vi "BStAT_(Singles) Update.vi"() -> ()   [LabVIEW 2014]
uses:
  <vilib>/vision/Image Controls.llb/IMAQ Image.ctl
  <vilib>/Utility/file.llb/Read From Spreadsheet File (string).vi
  <vilib>/Utility/file.llb/Read From Spreadsheet File (I64).vi
panel:
  out "Main tab 2":T1(ring)
  in  "fast rewind":bool
  out "refnum of data save file":refnum<file>
  in  "START":bool
  out "frames to write":i64[][](array[numeric])
  in  "Data file":path caption="Data"
  in  "playback speed":dbl(slide)=1.0 min=0.25 max=1.5 step=0.25 scale=0.25..1.5
  in  "Main tab":enum32{"Coding", "Display"}(tab)
  in  "Switch position":bool
  in  "Link Errors":bool
  in  "Player 2":bool
  in  "Player 1":bool
  in  "TC 3":bool
  in  "TR 3":bool
  in  "ML 3":bool
  in  "MC 3":bool
  in  "MR  3":bool
  in  "BC 3":bool
  in  "BL 3":bool
  in  "BR 3":bool
  in  "TL 3":bool
  in  "TC 2":bool
  in  "TR 2":bool
  in  "ML 2":bool
  in  "MC 2":bool
  in  "MR  2":bool
  in  "BC 2":bool
  in  "BL 2":bool
  in  "BR 2":bool
  in  "TL 2":bool
  in  "E2":bool
  in  "E1":bool
  in  "W2":bool
  in  "W1":bool
  in  "P2":i32
  in  "P1":i32
  in  "1 6":bool
  in  "2 6":bool
  in  "3 6":bool
  in  "4 6":bool
  in  "5 6":bool
  in  "6 6":bool
  in  "7 6":bool
  in  "8 6":bool
  in  "1 5":bool
  in  "2 5":bool
  in  "3 5":bool
  in  "4 5":bool
  in  "5 5":bool
  in  "6 5":bool
  in  "7 5":bool
  in  "8 5":bool
  in  "8 3":bool
  in  "7 3":bool
  in  "6 3":bool
  in  "5 3":bool
  in  "4 3":bool
  in  "3 3":bool
  in  "2 3":bool
  in  "1 3":bool
  in  "8 4":bool
  in  "7 4":bool
  in  "6 4":bool
  in  "5 4":bool
  in  "4 4":bool
  in  "3 4":bool
  in  "2 4":bool
  in  "1 4":bool
  in  "1 2":bool
  in  "2 2":bool
  in  "3 2":bool
  in  "4 2":bool
  in  "5 2":bool
  in  "6 2":bool
  in  "7 2":bool
  in  "8 2":bool
  in  "5":bool
  in  "6":bool
  in  "7":bool
  in  "8":bool
  in  "1":bool
  in  "2":bool
  in  "3":bool
  in  "4":bool
  in  "S1":bool
  in  "S2":bool
  in  "1 7":bool
  in  "2 7":bool
  in  "3 7":bool
  in  "4 7":bool
  in  "Code lag(s)":dbl=1.0 min=0.0 max=5.0 step=0.5 format="%#.1g"
  in  "Pause lag(s)":dbl=1.0 min=0.0 max=2.0 step=0.5 format="%#.1g"
  in  "Pause lag on":bool
  in  "Btn 5":string
  in  "Btn 4":string
  in  "Btn 3":string
  in  "Btn 2":string
  in  "Btn 1":string
  in  "Button 1":bool
  in  "Button 5":bool
  in  "Button 4":bool
  in  "Button 3":bool
  in  "Button 2":bool
  in  "Display tab":enum32{"Edit ", "Data Display", "Momentum"}(tab)
  in  "Combine":bool
  out "Btn 6":string
  out "Btn 7":string
  out "Btn 8":string
  out "Btn 9":string
  out "Btn 10":string
  in  "Button 6":bool
  in  "Button 10":bool
  in  "Button 9":bool
  in  "Button 8":bool
  in  "Button 7":bool
  in  "ST":bool
  in  "CR 2":bool
  in  "player2":bool
  in  "player1":bool
  in  "REPORT":bool
  out "Video files to write":string[](array[string])
  in  "Video compress":bool=TRUE
  in  "Abort":bool
  in  "Write file":bool
  in  "Delete":bool[](array[boolean])
  out "Writing":u32(slide) scale=0.0..51.0
  in  "File name":string
  in  "Add to lib":bool
  in  "Video to write":path caption="Folder"
  in  "Examine code":bool
  in  "Update":bool
  in  "Reset":bool
  in  "Code number display":i32 min=1 max=20
  in  "Next":bool
  in  "Previous":bool
  in  "lob":bool
  in  "clear":bool
  in  "drive":bool
  in  "smash":bool
  in  "defense":bool
  in  "chop":bool
  in  "drop":bool
  in  "net":bool
  in  "FH 2":bool
  in  "BH 2":bool
  in  "OH 2":bool
  in  "after":u8(slide)=2 scale=0.0..5.0
  in  "before":u8(slide)=2
  in  "point 2":bool
  in  "error":bool
  in  "winner":bool
  in  "point 1":bool
  in  "1 9":bool
  in  "service2":bool
  in  "service1":bool
  in  "2 9":bool
  in  "3 8":bool
  in  "4 8":bool
  in  "TL":bool
  in  "BR":bool
  in  "BL":bool
  in  "BM":bool
  in  "CR":bool
  in  "CM":bool
  in  "CL":bool
  in  "TR":bool
  in  "TM":bool
  in  "Extract data":bool
  in  "Upload edited video":bool
  in  "To make white":enum32{""}(tab)
  out "player12":string[](array[string])
  out "player2 2":string[](array[string])
  out "P1graph":cluster{dbl[], "array":dbl[]}(graph)={[0.0, nan, 0.0, nan, 0.0, nan, 0.0, nan, 0.0, nan, 0.0, nan, 0.0, nan, 0.0, nan, 0.0], "array"=[1.0, 2.0, 3.0, 4.0, 5.0, 6.0, 7.0, 8.0, 9.0, 10.0, 11.0, 12.0, 13.0, 14.0, 15.0, 16.0, 17.0]}
  out "P2graph":cluster{dbl[], "array":dbl[]}(graph)={[0.0, nan, 0.0, nan, 0.0, nan, 0.0, nan, 0.0, nan, 0.0, nan, 0.0, nan, 0.0, nan, 0.0], "array"=[1.0, 2.0, 3.0, 4.0, 5.0, 6.0, 7.0, 8.0, 9.0, 10.0, 11.0, 12.0, 13.0, 14.0, 15.0, 16.0, 17.0]}
  out "W1/E1":string[](array[string])
  out "W2/E2":string[](array[string])
  out "W/E2":string[](array[string])=["Fore hand", "Back hand", "Over head", "", "Strainght", "Cross", "", "Lob", "Clear", "Drive", "Smash", "Defence", "Chop", "Drop", "Net"]
  out "W/E1":string[](array[string])=["Fore hand", "Back hand", "Over head", "", "Strainght", "Cross", "", "Lob", "Clear", "Drive", "Smash", "Defence", "Chop", "Drop", "Net"]
  out "player2_2":string[](array[string])
  out "player1_2":string[](array[string])
  out "Player 4":string[](array[string])=["Fore hand", "Back hand", "Over head", "", "Straight", "Cross", "", "Smash", "Defense", "Drive/Tap", "Lob", "Drop", "Chop", "Clear", "Net"]
  out "Player 2_2":string[](array[string])=["Fore hand", "Back hand", "Over head", "", "Strainght", "Cross", "", "Lob", "Clear", "Drive", "Smash", "Defence", "Chop", "Drop", "Net"]
  out "Player 1_2":string[](array[string])=["Fore hand", "Back hand", "Over head", "", "Strainght", "Cross", "", "Lob", "Clear", "Drive", "Smash", "Defence", "Chop", "Drop", "Net"]
  out "Player 3":string[](array[string])=["Fore hand", "Back hand", "Over head", "", "Straight", "Cross", "", "Smash", "Defense", "Drive/Tap", "Lob", "Drop", "Chop", "Clear", "Net"]
  out "p2 17":string
  out "p2 16":string
  out "p2 11":string
  out "p2 10":string
  out "p2 9":string
  out "p2 14":string
  out "p2 13":string
  out "p2 12":string
  out "p2 15":string
  out "p1 5":string
  out "p1 7":string
  out "p1 6":string
  out "p1 4":string
  out "p1 1":string
  out "p1 3":string
  out "p1 2":string
  out "p1 8":string
  out "p1 9":string
  in  "save2":string
  in  "save1":string
  in  "save2 3":bool
  in  "save1 3":bool
  in  "Compare":bool
  in  "2 8":string(combo)="1"
  in  "1 8":string(combo)="1"
  in  "display\nselection":string(combo)="1"
  in  "Percentage":bool
  in  "to make white 2":enum32{""}(tab)
  out "Shortest rally length(sec)":dbl format="%#_3g"
  out "Longest rally length(sec)":dbl format="%#_3g"
  out "Score":dbl[](array[numeric])
  out "Average rally length(sec)":dbl format="%#_3g"
  out "Rally length(sec)":dbl format="%#_3g"
  out "momentum graph":cluster{dbl[], dbl[]}[](graph)
  in  "Load video":bool
  in  "Play":bool
  out "ful video frames":i64[](array[numeric])
  out "playback speed":dbl
  out "Number of Frames":u32
  out "framesPerSecond":u32
  out "Last Edit":bool[](array[boolean])
  out "frames 2 play":i64[](array[numeric])
  in  "stop":bool
  out "Video Frame":u32
  out "save1 2":i32[][](array[numeric])
  out "save1_data":dbl[][](array[numeric])
  out "save2 2":i32[][](array[numeric])
  out "save2_data":dbl[][](array[numeric])
  out "game":i32[][](array[numeric])
  out "comp_p1":dbl[](array[numeric])
  out "comp_p2":dbl[](array[numeric])
  out "comp_p2 2":dbl[](array[numeric])
  out "comp_p1 2":dbl[](array[numeric])
  out "Score 2":i64[][](array[numeric])
  out "frame data":i64[][](array[numeric])
  out "coded data":i64[][](array[numeric])
  out "edited\nevents":i64[][](array[numeric])
  out "edited to play":i64[](array[numeric])
  out "frames edited":i64[](array[numeric])
  out "service frames":i64[](array[numeric])
  out "point frames":i64[](array[numeric])
  out "p1y":dbl[](array[numeric])
  out "p2y":dbl[](array[numeric])
  in  "fast forward":bool
  in  "Pause":bool
  out "coding":i64[][](array[numeric])
  out "FH":bool[](array[boolean])
  out "BH":bool[](array[boolean])
  out "OH":bool[](array[boolean])
  out "P1 position":bool
  out "P2 position":bool
  in  "Progress...":u32(slide) min=400 max=47374 scale=-1.1..47173.0
  in  "Video file":path caption="Video"
  out "task":i32(slide) scale=0.0..300.0
  out "Video":T2(plugin-control)
  # "Strategic Analysis Tool for Badminton"
  # "© 2012 National Sports Institute of Malaysia All Rights Reserved"
  # "Position"
  # "Rally start"
  # "Rally end"
  # "Switch sides"
  # "Smash"
  # "Defence"
  # "Drive/Tap"
  # "Lob"
  # "Drop"
  # "Chop"
  # "Clear"
  # "Net"
  # "Forehand"
  # "Backhand"
  # "Overhead"
  # "Straight"
  # "Cross"
  # "Straight"
  # "Cross"
  # "Straight"
  # "Cross"
  # "Shots"
  # "Custom coding"
  # "Playback interval (s)"
  # "Rally end"
  # "Rally start"
  # "Position"
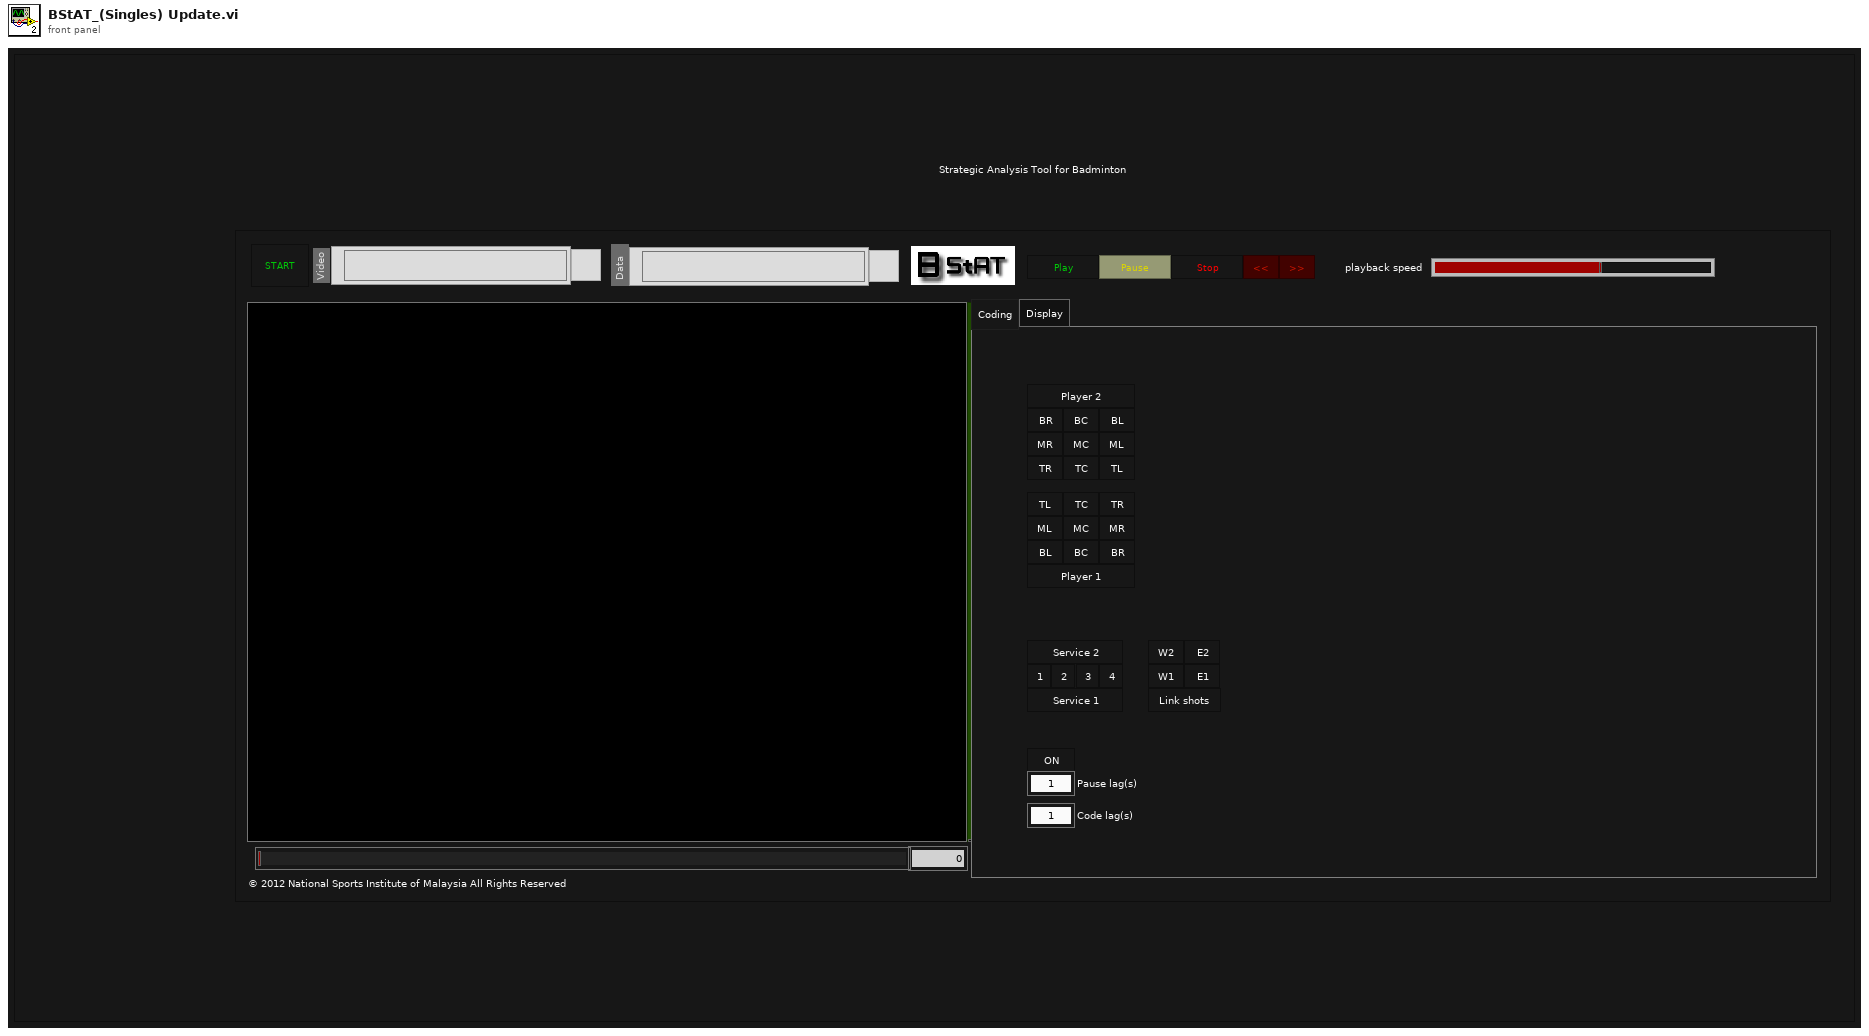
[diagram p1: front panel]
types:
  T1 = enum32{"Coding", "Edit video", "Examine coding", "Display", "Update coding", "Edit coding"}
  T2 = typedef "IMAQ Image.ctl" = refnum<image>
  T3 = enum16{"open", "replace", "create", "open or create", "replace or create", "replace or create with confirmation"}
  T4 = enum8{"Enabled", "Disabled", "Disabled and Grayed Out"}
  T5 = typedef "Image Type" = u32
  T6 = typedef "AviRefnum.ctl" = refnum<k1>
  T7 = cluster{"width":u32, "height":u32, "framesPerSecond":u32, "compressionFilter":string, "hasData":bool}
  T8 = typedef "LVPositionTypeDef.ctl" = cluster{"Left":i32, "Top":i32}
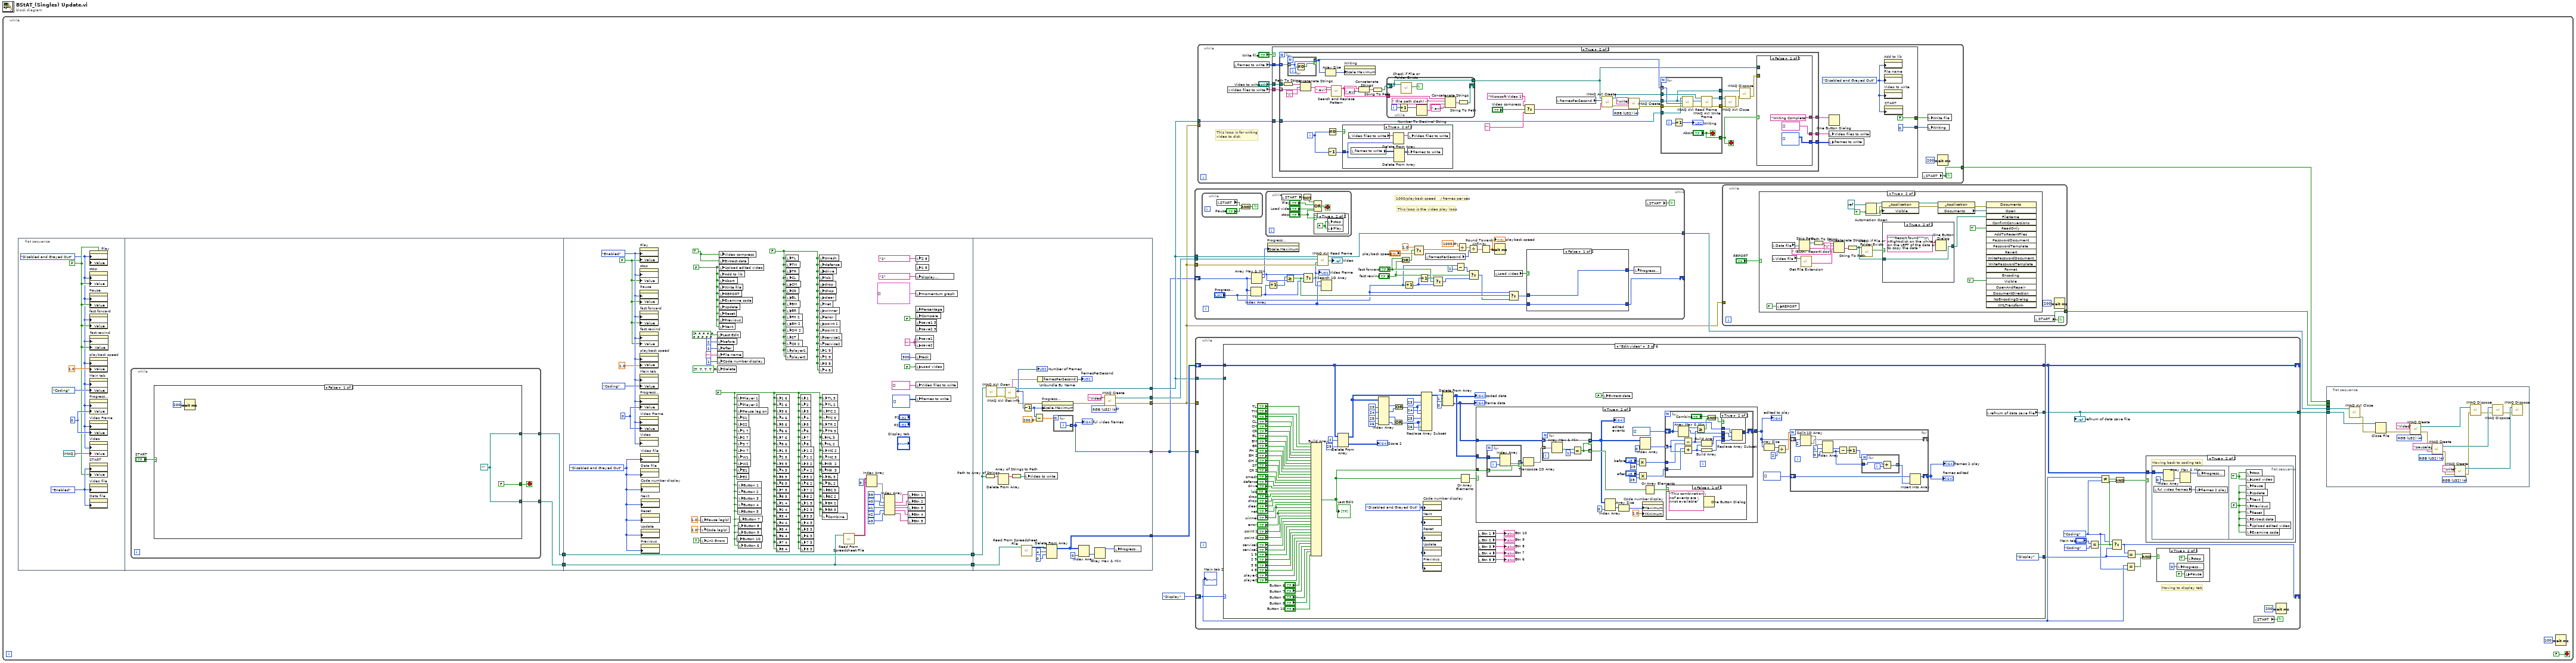
[diagram p0: block diagram]
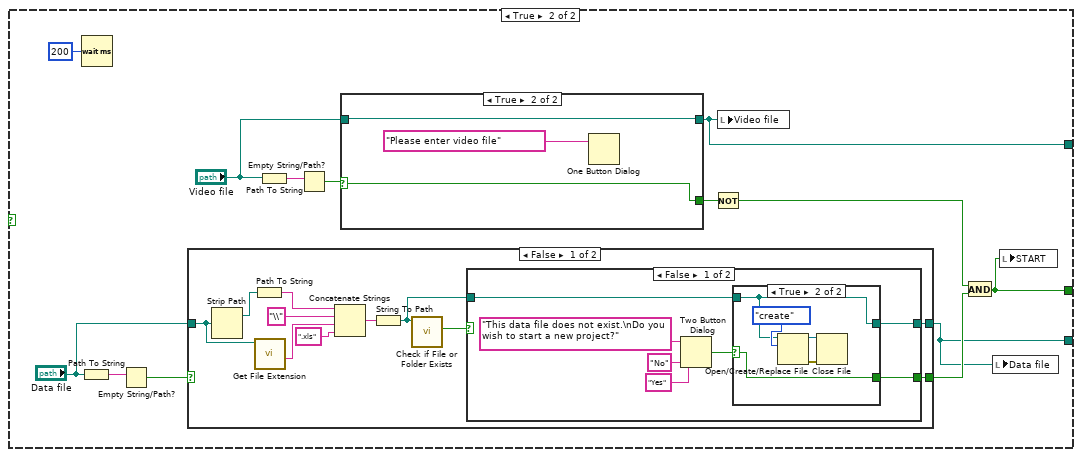
[diagram p2: hidden frame]
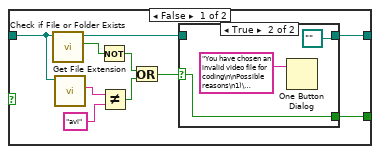
[diagram p3: hidden frame]
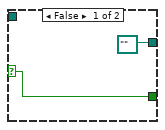
[diagram p5: hidden frame]
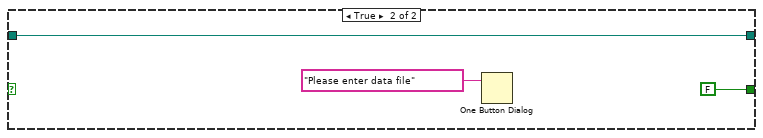
[diagram p7: hidden frame]
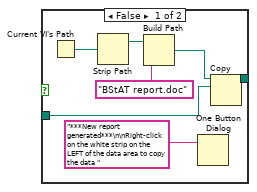
[diagram p9: hidden frame]
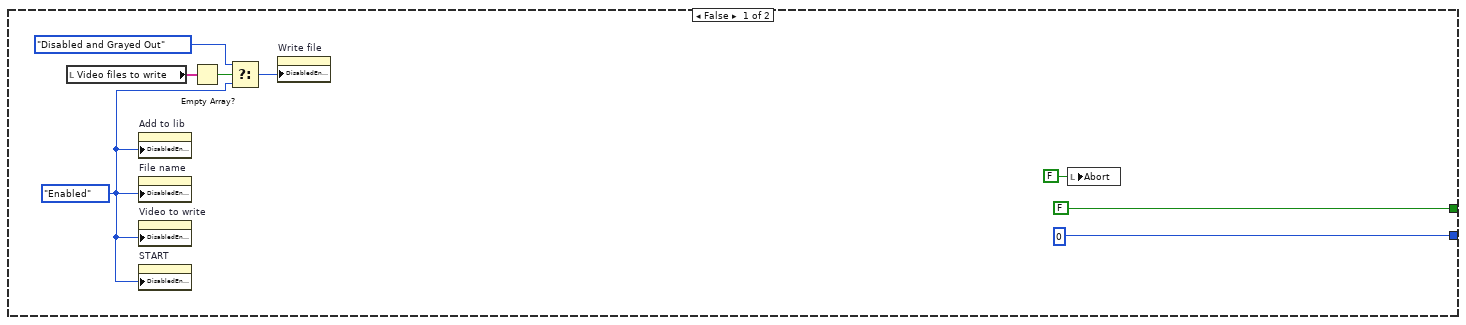
[diagram p10: hidden frame]
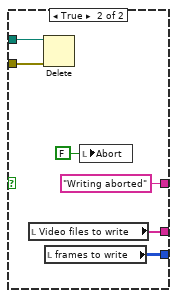
[diagram p11: hidden frame]
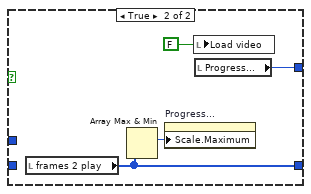
[diagram p14: hidden frame]
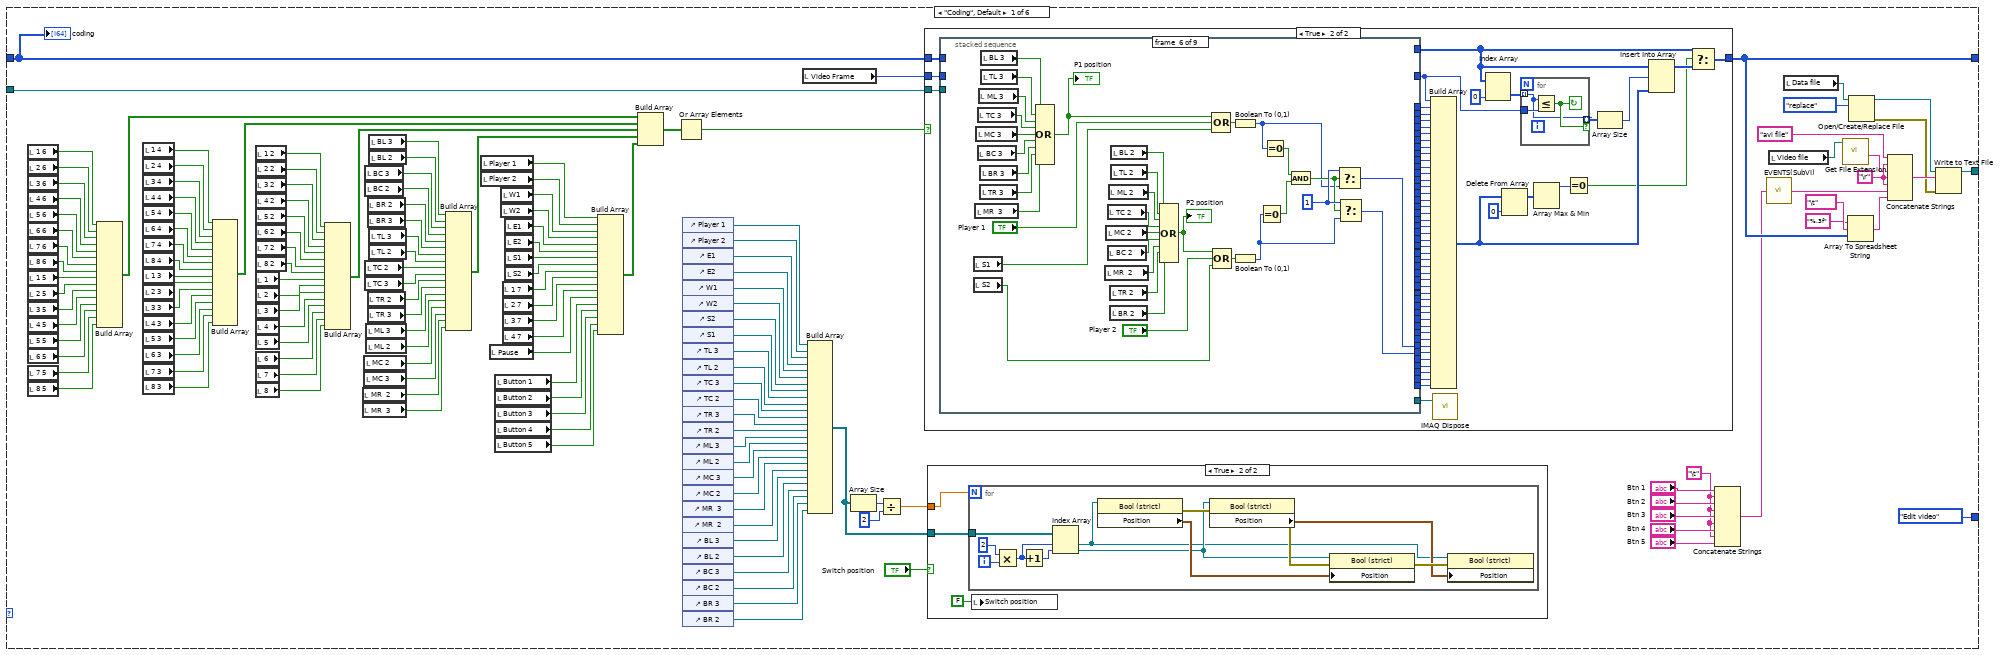
[diagram p17: hidden frame]
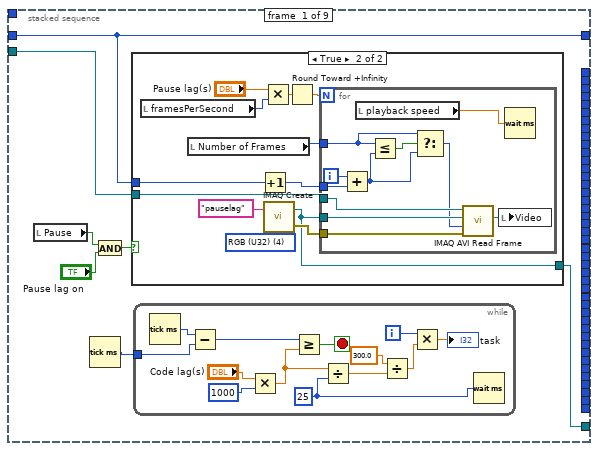
[diagram p20: hidden frame]
diagram:
  n1 = while {
    stop <- FALSE stop-if-true
    n2 = flat-sequence {
      tunnel: [w42] -> w15
      tunnel: [w43] -> w16
      tunnel: w16 -> [w128]
      tunnel: w15 -> [w127]
      tunnel: [w127] -> w14
      tunnel: [w128] -> w13
      tunnel: w14 -> [w176]
      tunnel: w13 -> [w159]
      tunnel: [w175] -> w11
      tunnel: [w158] -> w10
      tunnel: [w157] -> w9
      tunnel: [w156] -> w1
      tunnel: [w155] -> w8
      frame #0 {
        w37 = T4."Enabled" ("Disabled")
        w39 = u32 0 ("Progress...")
        w36 = FALSE ("START")
        w35 = T4."Disabled and Grayed Out" ("Disabled")
        n3 = property on="Play" class="Bool (strict)"("DisabledEnum"=w35, "Value"=w36) -> ()  [unwired: 2 in, 2 out]
        n4 = property on="stop" class="Bool (strict)"("DisabledEnum"=w35, "Value"=w36) -> ()  [unwired: 2 in, 2 out]
        n5 = property on="Pause" class="Bool (strict)"("DisabledEnum"=w35, "Value"=w36) -> ()  [unwired: 2 in, 2 out]
        n6 = property on="fast forward" class="Bool (strict)"("DisabledEnum"=w35, "Value"=w36) -> ()  [unwired: 2 in, 2 out]
        n7 = property on="playback speed" class="Slide (strict)"("DisabledEnum"=w35, "Value"=1.0 ("playback speed")) -> ()  [unwired: 2 in, 2 out]
        n8 = property on="Main tab" class="TabCtl (strict)"("DisabledEnum"=w35, "Value"=enum32{"Coding", "Display"}."Coding" ("Main tab")) -> ()  [unwired: 2 in, 2 out]
        n9 = property on="Progress..." class="Slide (strict)"("DisabledEnum"=w35, "Value"=w39) -> ()  [unwired: 2 in, 2 out]
        n10 = property on="Video Frame" class="DigNum (strict)"("DisabledEnum"=w35, "Value"=w39) -> ()  [unwired: 2 in, 2 out]
        n11 = property on="Video" class="ImageControl"("DisabledEnum"=w35, "Value"=T2 refnum ("Video")) -> ()  [unwired: 2 in, 2 out]
        n12 = property on="START" class="Bool (strict)"("DisabledEnum"=w37, "Value"=w36) -> ()  [unwired: 2 in, 2 out]
        n13 = property on="Video file" class="Path"("DisabledEnum"=w37) -> ()  [unwired: 2 in, 2 out]
        n14 = property on="Data file" class="Path"("DisabledEnum"=w37) -> ()  [unwired: 2 in, 2 out]
        n15 = property on="fast rewind" class="Bool (strict)"("DisabledEnum"=w35, "Value"=w36) -> ()  [unwired: 2 in, 2 out]
      }
      frame #1 {
        n16 = while {
          tunnel: [w45] -> w43
          tunnel: [w44] -> w42
          stop <- w46 stop-if-true
          n17 = case shown="False" "START" {
            tunnel: [FALSE w51] -> w46
            tunnel: [w48 w54] -> w45
            tunnel: [w48 w53] -> w44
            frame False {
              w48 = path "" ("dup path")
              n18 = Wait (ms)(milliseconds to wait=u32 200) -> ()  [unwired: 1 out]
            }
            frame True {
              n19 = Path To String(path="Data file") -> (string=w63:string)
              n20 = Wait (ms)(milliseconds to wait=u32 200) -> ()  [unwired: 1 out]
              n21 = Empty String/Path?(string/path=w63) -> (empty?=w62:bool)
              n22 = case shown="False" w62 {
                tunnel: "Data file" -> [w84 w109]
                tunnel: [w83 FALSE] -> w60
                tunnel: [w82 w109] -> w53
                frame False {
                  n23 = Strip Path(path=w84) -> (stripped path=w89:path)  [unwired: 1 out]
                  n24 = Path To String(path=w89) -> (string=w88:string)
                  n25 = call <vilib>:"Get File Extension.vi"("file"=w84) -> ("filename without extension"=w91:string)  [unwired: 7 in, 3 out]
                  n26 = Concatenate Strings(w88, "\\" ("string"), w91, ".xls" ("string")) -> (w90:string)
                  n27 = String To Path(string=w90) -> (path=w85:path)
                  n28 = call <vilib>:"Check if File or Folder Exists.vi"("path"=w85) -> ("file or folder exists?"=w86:bool)  [unwired: 8 in, 2 out]
                  n29 = case shown="False" w86 {
                    selector: w86 -> [_ w108]
                    tunnel: w85 -> [w95 w107]
                    tunnel: [w94 w108] -> w83
                    tunnel: [w93 w107] -> w82
                    frame False {
                      n30 = Two Button Dialog(message="This data file does not exist.\nDo you wish to start a new project?", 1:"No" ("F button name (\"Cancel\")"), 2:"Yes" ("T button name (\"OK\")")) -> (T button?=w96:bool)
                      n31 = case shown="True" w96 {
                        selector: w96 -> [w101 w103]
                        tunnel: w95 -> [_ w102]
                        tunnel: [w101 w103] -> w94
                        tunnel: [path "" ("dup path") w102] -> w93
                        frame False {
                        }
                        frame True {
                          n32 = Open/Create/Replace File(file path (use dialog)=w102, operation (0:open)=T3."create") -> (refnum out=w104:refnum<file>, error out=w106:errorcluster)  [unwired: 4 in, 1 out]
                          n33 = Close File(refnum=w104, error in=w106) -> ()  [unwired: 2 out]
                        }
                      }
                    }
                    frame True {
                    }
                  }
                }
                frame True {
                  n34 = One Button Dialog(message="Please enter data file") -> ()  [unwired: 1 in, 1 out]
                }
              }
              n35 = Path To String(path="Video file") -> (string=w58:string)
              n36 = Empty String/Path?(string/path=w58) -> (empty?=w57:bool)
              n37 = case shown="True" w57 {
                selector: w57 -> [_ w81]
                tunnel: "Video file" -> [w68 w79]
                tunnel: [w65 w79] -> w54
                tunnel: [w64 w81] -> w55
                frame False {
                  n38 = call <vilib>:"Check if File or Folder Exists.vi"("path"=w68) -> ("file or folder exists?"=w72:bool, "dup path"=w66:path)  [unwired: 8 in, 1 out]
                  n39 = call <vilib>:"Get File Extension.vi"("file"=w68) -> ("lowercase file extension"=w69:string)  [unwired: 7 in, 3 out]
                  n40 = Not(x=w72) -> (.not. x?=w73:bool)
                  n41 = Not Equal?(x=w69, y="avi" ("lowercase file extension")) -> (x != y?=w71:bool)
                  n42 = Or(x=w73, y=w71) -> (x .or. y?=w67:bool)
                  n43 = case shown="True" w67 {
                    selector: w67 -> [w74 w76]
                    tunnel: w66 -> [w75 _]
                    tunnel: [w75 path "" ("dup path")] -> w65
                    tunnel: [w74 w76] -> w64
                    frame False {
                    }
                    frame True {
                      n44 = One Button Dialog(message="You have chosen an invalid video file for coding\n\nPossible reasons\n1)\tChosen video file format was not AVI\n2)\tChosen video file does not exist") -> ()  [unwired: 1 in, 1 out]
                    }
                  }
                }
                frame True {
                  n45 = One Button Dialog(message="Please enter video file") -> ()  [unwired: 1 in, 1 out]
                }
              }
              n46 = Not(x=w55) -> (.not. x?=w59:bool)
              n47 = local write "Video file"(w54) -> ()
              n48 = And(x=w59, y=w60) -> (x .and. y?=w51:bool)
              n49 = local write "Data file"(w53) -> ()
              n50 = local write "START"(w51) -> ()
            }
          }
        }
      }
      frame #2 {
        w136 = "" ("save2")
        w137 = "1" ("2 8")
        w140 = FALSE ("4 6")
        w113 = FALSE ("4 6")
        w151 = FALSE ("4 6")
        w149 = FALSE ("4 6")
        w148 = TRUE ("Extract data")
        w112 = T4."Disabled and Grayed Out" ("Disabled")
        w154 = u32 0 ("Progress...")
        w129 = FALSE ("START")
        w130 = T4."Enabled" ("Disabled")
        n51 = property on="Play" class="Bool (strict)"("DisabledEnum"=w130, "Value"=w129) -> ()  [unwired: 2 in, 2 out]
        n52 = property on="stop" class="Bool (strict)"("DisabledEnum"=w130, "Value"=w129) -> ()  [unwired: 2 in, 2 out]
        n53 = property on="Pause" class="Bool (strict)"("DisabledEnum"=w130, "Value"=w129) -> ()  [unwired: 2 in, 2 out]
        n54 = property on="fast forward" class="Bool (strict)"("DisabledEnum"=w130, "Value"=w129) -> ()  [unwired: 2 in, 2 out]
        n55 = property on="fast rewind" class="Bool (strict)"("DisabledEnum"=w130, "Value"=w129) -> ()  [unwired: 2 in, 2 out]
        n56 = property on="playback speed" class="Slide (strict)"("DisabledEnum"=w130, "Value"=1.0 ("playback speed")) -> ()  [unwired: 2 in, 2 out]
        n57 = property on="Main tab" class="TabCtl (strict)"("DisabledEnum"=w130, "Value"=enum32{"Coding", "Display"}."Coding" ("Main tab")) -> ()  [unwired: 2 in, 2 out]
        n58 = property on="Progress..." class="Slide (strict)"("DisabledEnum"=w130, "Value"=w154) -> ()  [unwired: 2 in, 2 out]
        n59 = property on="Video Frame" class="DigNum (strict)"("DisabledEnum"=w130, "Value"=w154) -> ()  [unwired: 2 in, 2 out]
        n60 = property on="Video" class="ImageControl"("DisabledEnum"=w130) -> ()  [unwired: 2 in, 2 out]
        n61 = property on="Video file" class="Path"("DisabledEnum"=w112) -> ()  [unwired: 2 in, 2 out]
        n62 = property on="Data file" class="Path"("DisabledEnum"=w112) -> ()  [unwired: 2 in, 2 out]
        n63 = property on="Code number display" class="DigNum (strict)"("DisabledEnum"=w112) -> ()  [unwired: 2 in, 2 out]
        n64 = property on="Next" class="Bool (strict)"("DisabledEnum"=w112) -> ()  [unwired: 2 in, 2 out]
        n65 = property on="Reset" class="Bool (strict)"("DisabledEnum"=w112) -> ()  [unwired: 2 in, 2 out]
        n66 = property on="Update" class="Bool (strict)"("DisabledEnum"=w112) -> ()  [unwired: 2 in, 2 out]
        n67 = property on="Previous" class="Bool (strict)"("DisabledEnum"=w112) -> ()  [unwired: 2 in, 2 out]
        n68 = local write "Pause lag(s)"(1.0 ("Pause lag(s)")) -> ()
        n69 = local write "Code lag(s)"(2.0 ("Code lag(s)")) -> ()
        n70 = local write "Link Errors"(TRUE ("Link Errors")) -> ()
        n71 = local write "Last Edit"(bool[] [FALSE, FALSE, FALSE, FALSE, FALSE, FALSE, FALSE, FALSE, FALSE, FALSE, FALSE, FALSE, FALSE, FALSE, FALSE, FALSE, FALSE, FALSE, FALSE, FALSE, FALSE, FALSE, FALSE, FALSE, FALSE, FALSE, FALSE, FALSE, FALSE, FALSE, FALSE, FALSE, FALSE, FALSE, FALSE, FALSE] ("Last Edit")) -> ()
        n72 = local write "before"(u8 2 ("before")) -> ()
        n73 = local write "after"(u8 2 ("after")) -> ()
        n74 = local write "File name"("" ("File name")) -> ()
        n75 = local write "Code number display"(1 ("Code number display")) -> ()
        n76 = local write "Delete"(bool[] [TRUE, TRUE, TRUE, TRUE, TRUE] ("Array 2")) -> ()
        n77 = local write "Video compress"(w148) -> ()
        n78 = local write "Extract data"(w148) -> ()
        n79 = local write "Upload edited video"(w151) -> ()
        n80 = local write "Add to lib"(w151) -> ()
        n81 = local write "Abort"(w151) -> ()
        n82 = local write "Write file"(w151) -> ()
        n83 = local write "REPORT"(w151) -> ()
        n84 = local write "Examine code"(w151) -> ()
        n85 = local write "Update"(w151) -> ()
        n86 = local write "Reset"(w151) -> ()
        n87 = local write "Previous"(w151) -> ()
        n88 = local write "Next"(w151) -> ()
        n89 = local write "Player 1"(w113) -> ()
        n90 = local write "Player 2"(w113) -> ()
        n91 = local write "Pause lag on"(w113) -> ()
        n92 = local write "S1"(w113) -> ()
        n93 = local write "S2"(w113) -> ()
        n94 = local write "1 7"(w113) -> ()
        n95 = local write "2 7"(w113) -> ()
        n96 = local write "3 7"(w113) -> ()
        n97 = local write "4 7"(w113) -> ()
        n98 = local write "W1"(w113) -> ()
        n99 = local write "W2"(w113) -> ()
        n100 = local write "E1"(w113) -> ()
        n101 = local write "E2"(w113) -> ()
        n102 = local write "Button 10"(w113) -> ()
        n103 = local write "Button 1"(w113) -> ()
        n104 = local write "Button 2"(w113) -> ()
        n105 = local write "Button 3"(w113) -> ()
        n106 = local write "Button 4"(w113) -> ()
        n107 = local write "Button 5"(w113) -> ()
        n108 = local write "Button 8"(w113) -> ()
        n109 = local write "Button 9"(w113) -> ()
        n110 = local write "Button 6"(w113) -> ()
        n111 = local write "Button 7"(w113) -> ()
        n112 = local write "1 6"(w113) -> ()
        n113 = local write "2 6"(w113) -> ()
        n114 = local write "3 6"(w113) -> ()
        n115 = local write "4 6"(w113) -> ()
        n116 = local write "5 6"(w113) -> ()
        n117 = local write "6 6"(w113) -> ()
        n118 = local write "7 6"(w113) -> ()
        n119 = local write "8 6"(w113) -> ()
        n120 = local write "1 5"(w113) -> ()
        n121 = local write "2 5"(w113) -> ()
        n122 = local write "3 5"(w113) -> ()
        n123 = local write "4 5"(w113) -> ()
        n124 = local write "5 5"(w113) -> ()
        n125 = local write "6 5"(w113) -> ()
        n126 = local write "7 5"(w113) -> ()
        n127 = local write "8 5"(w113) -> ()
        n128 = local write "1 4"(w113) -> ()
        n129 = local write "2 4"(w113) -> ()
        n130 = local write "3 4"(w113) -> ()
        n131 = local write "4 4"(w113) -> ()
        n132 = local write "5 4"(w113) -> ()
        n133 = local write "6 4"(w113) -> ()
        n134 = local write "7 4"(w113) -> ()
        n135 = local write "8 4"(w113) -> ()
        n136 = local write "TL"(w149) -> ()
        n137 = local write "TM"(w149) -> ()
        n138 = local write "TR"(w149) -> ()
        n139 = local write "CL"(w149) -> ()
        n140 = local write "CM"(w149) -> ()
        n141 = local write "CR"(w149) -> ()
        n142 = local write "BL"(w149) -> ()
        n143 = local write "BM"(w149) -> ()
        n144 = local write "BR"(w149) -> ()
        n145 = local write "FH 2"(w149) -> ()
        n146 = local write "BH 2"(w149) -> ()
        n147 = local write "OH 2"(w149) -> ()
        n148 = local write "ST"(w149) -> ()
        n149 = local write "CR 2"(w149) -> ()
        n150 = local write "player1"(w149) -> ()
        n151 = local write "player2"(w149) -> ()
        n152 = local write "1"(w113) -> ()
        n153 = local write "2"(w113) -> ()
        n154 = local write "3"(w113) -> ()
        n155 = local write "4"(w113) -> ()
        n156 = local write "5"(w113) -> ()
        n157 = local write "6"(w113) -> ()
        n158 = local write "7"(w113) -> ()
        n159 = local write "8"(w113) -> ()
        n160 = local write "1 2"(w113) -> ()
        n161 = local write "2 2"(w113) -> ()
        n162 = local write "3 2"(w113) -> ()
        n163 = local write "4 2"(w113) -> ()
        n164 = local write "5 2"(w113) -> ()
        n165 = local write "6 2"(w113) -> ()
        n166 = local write "7 2"(w113) -> ()
        n167 = local write "8 2"(w113) -> ()
        n168 = local write "1 3"(w113) -> ()
        n169 = local write "2 3"(w113) -> ()
        n170 = local write "3 3"(w113) -> ()
        n171 = local write "4 3"(w113) -> ()
        n172 = local write "5 3"(w113) -> ()
        n173 = local write "6 3"(w113) -> ()
        n174 = local write "7 3"(w113) -> ()
        n175 = local write "8 3"(w113) -> ()
        n176 = local write "smash"(w149) -> ()
        n177 = local write "defense"(w149) -> ()
        n178 = local write "drive"(w149) -> ()
        n179 = local write "lob"(w149) -> ()
        n180 = local write "drop"(w149) -> ()
        n181 = local write "chop"(w149) -> ()
        n182 = local write "clear"(w149) -> ()
        n183 = local write "net"(w149) -> ()
        n184 = local write "winner"(w149) -> ()
        n185 = local write "error"(w149) -> ()
        n186 = local write "point 1"(w149) -> ()
        n187 = local write "point 2"(w149) -> ()
        n188 = local write "service1"(w149) -> ()
        n189 = local write "service2"(w149) -> ()
        n190 = local write "1 9"(w149) -> ()
        n191 = local write "2 9"(w149) -> ()
        n192 = local write "3 8"(w149) -> ()
        n193 = local write "4 8"(w149) -> ()
        n194 = local write "ML 3"(w113) -> ()
        n195 = local write "ML 2"(w113) -> ()
        n196 = local write "MR  2"(w113) -> ()
        n197 = local write "MR  3"(w113) -> ()
        n198 = local write "TL 3"(w113) -> ()
        n199 = local write "TL 2"(w113) -> ()
        n200 = local write "TR 2"(w113) -> ()
        n201 = local write "TR 3"(w113) -> ()
        n202 = local write "MC 2"(w113) -> ()
        n203 = local write "MC 3"(w113) -> ()
        n204 = local write "BL 3"(w113) -> ()
        n205 = local write "BL 2"(w113) -> ()
        n206 = local write "BR 2"(w113) -> ()
        n207 = local write "BR 3"(w113) -> ()
        n208 = local write "TC 2"(w113) -> ()
        n209 = local write "TC 3"(w113) -> ()
        n210 = local write "BC 3"(w113) -> ()
        n211 = local write "BC 2"(w113) -> ()
        n212 = local write "Combine"(w113) -> ()
        n213 = call-poly <vilib>:"Read From Spreadsheet File.vi"("file path (dialog if empty)"=w127) -> ("all rows"=w126:string[][])  [unwired: 6 in, 4 out]
        n214 = Index Array(array=w126, index (row)=3) -> (element=w124:string[])  [unwired: 1 in]
        n215 = Index Array(array=w124, index #1=39 ("index"), index #2=40 ("index"), index #3=41 ("index"), index #4=42 ("index"), index #5=43 ("index")) -> (element #1=w118:string, element #2=w117:string, element #3=w116:string, element #4=w115:string, element #5=w114:string)
        n216 = local write "Btn 1"(w118) -> ()
        n217 = local write "Btn 2"(w117) -> ()
        n218 = local write "Btn 3"(w116) -> ()
        n219 = local write "Btn 4"(w115) -> ()
        n220 = local write "Btn 5"(w114) -> ()
        n221 = local write "2 8"(w137) -> ()
        n222 = local write "1 8"(w137) -> ()
        n223 = local write "display\nselection"("1" ("display\nselection")) -> ()
        n224 = local write "momentum graph"(cluster{dbl[], dbl[]}[] [] ("momentum graph")) -> ()
        n225 = local write "Percentage"(w140) -> ()
        n226 = local write "Compare"(w140) -> ()
        n227 = local write "save1 3"(w140) -> ()
        n228 = local write "save2 3"(w140) -> ()
        n229 = local write "save1"(w136) -> ()
        n230 = local write "save2"(w136) -> ()
        n231 = local write "task"(300 ("task")) -> ()
        n232 = local write "Load video"(FALSE ("Pause")) -> ()
        n233 = local write "Video files to write"(string[] [] ("Video files to write")) -> ()
        n234 = local write "frames to write"(i64[][] [] ("to write")) -> ()
      }
      frame #3 {
        w161 = T5 4 items=["Grayscale (U8)", "Grayscale (I16)", "Grayscale (SGL)", "Complex (CSG)", "RGB (U32)", "HSL (U32)", "RGB (U64)"] ("Image Type")
        n235 = Path to Array of Strings(0:w159) -> (2:w172:string[])  [unwired: 1 out]
        n236 = call "IMAQ AVI Open"("AVI Path"=w159) -> ("error out"=w163:errorcluster, "Avi Refnum"=w162:T6)  [unwired: 9 in]
        n237 = Delete From Array(array=w172) -> (array with subset deleted=w173:string[])  [unwired: 2 in, 1 out]
        n238 = call "IMAQ AVI Get Info"("error in (no error)"=w163, "Avi Refnum"=w162) -> ("error out"=w165:errorcluster, "Number of Frames"=w168:u32, "Avi Refnum (duplicate)"=w158:T6, "Frame Data"=w164:T7)  [unwired: 5 in, 1 out]
        "Number of Frames" <- w168
        n239 = Array of Strings to Path(0:w173) -> (2:w174:path)  [unwired: 1 in]
        n240 = call-poly <vilib>:"Read From Spreadsheet File.vi"("file path (dialog if empty)"=w176) -> ("all rows"=w179:i64[][])  [unwired: 6 in, 4 out]
        n241 = Decrement(x=w168) -> (x-1=w171:u32)
        n242 = local write "Video to write"(w174) -> ()
        n243 = Subtract(x=w171, y=200.0) -> (x-y=w169:dbl)
        n244 = Unbundle By Name(w164) -> ("framesPerSecond"=→"framesPerSecond":u32)
        n245 = property on="Progress..." class="Slide (strict)"(error in=w165, "Scale.Maximum"=w171) -> (error out=w166:errorcluster)  [unwired: 1 in, 1 out]
        n246 = Delete From Array(array=w179, length=4, index (row)=0) -> (array with subset deleted=w175:i64[][])  [unwired: 1 in, 1 out]
        n247 = for {
          N: w169 -> [_]
          tunnel: [w183] -> w155 mode=indexing
          i -> [w183]
        }
        "ful video frames" <- w155
        n248 = Index Array(array=w175, index (col)=0 ("disabled index (col)")) -> (element=w181:i64[])  [unwired: 1 in]
        n249 = Array Max & Min(array=w181) -> (max value=w180:i64)  [unwired: 3 out]
        n250 = call "IMAQ Create"("Image Name"="Video", "Image Type"=w161, "error in (no error)"=w166) -> ("New Image"=w157:T2, "error out"=w156:errorcluster)  [unwired: 2 in]
        n251 = local write "Progress..."(w180) -> ()
      }
    }
    n252 = while {
      tunnel: w10 -> [w355]
      tunnel: w9 -> [w354]
      tunnel: w1 -> [w353]
      shift-right: [w347] -> _
      shift-left: w8 -> [w346]
      tunnel: [w330] -> w4
      stop <- w331 continue-if-true
      # "This loop is the video play loop"
      # "1000/playback speed    / frames per sec"
      n253 = while {
        stop <- w371 continue-if-true
        n254 = local read "START"() -> (w370:bool)
        n255 = And(x=w370, y="Pause") -> (x .and. y?=w371:bool)
      }
      n256 = Index Array(array=w346, index="Progress...") -> (element=w333:i64)
      n257 = Array Max & Min(array=w346) -> (max value=w351:i64, max index (indices)=w352:i32)  [unwired: 2 out]
      n258 = while {
        stop <- w360 stop-if-true
        n259 = local read "START"() -> (w357:bool)
        n260 = Not(x=w357) -> (.not. x?=w356:bool)
        n261 = Compound Arithmetic op=OR(w356, "Play", "Load video", "stop") -> (w360:bool)
        n262 = case shown="True" "stop" {
          frame False {
          }
          frame True {
            w362 = FALSE ("Play")
            n263 = local write "stop"(w362) -> ()
            n264 = local write "Play"(w362) -> ()
          }
        }
      }
      n265 = property on="Progress..." class="Slide (strict)"("Scale.Maximum"=w352) -> ()  [unwired: 2 in, 2 out]
      n266 = Increment(x=w333) -> (x+1=w334:i64)
      n267 = Greater Or Equal?(x=w334, y=w351) -> (x >= y?=w337:bool)
      n268 = Select(t=w351, s=w337, f=w333) -> (s? t:f=w348:i64)
      "Video Frame" <- w348
      n269 = call "IMAQ AVI Read Frame"("error in (no error)"=w353, "Frame Number"=w348, "Image"=w354, "Avi Refnum"=w355) -> ("Image Out"=→"Video":T2, "Avi Refnum (duplicate)"=w330:T6)  [unwired: 4 in, 2 out]
      n270 = Search 1D Array(1D array=w346, element=w348) -> ()  [unwired: 1 in, 1 out]
      n271 = Or(x="fast forward", y="fast rewind") -> (x .or. y?=w328:bool)
      n272 = Increment(x="Progress...") -> (x+1=w329:u32)
      n273 = Select(t=1.0, s=w328, f="playback speed") -> (s? t:f=w340:dbl)
      n274 = Increment(x=w329) -> (x+1=w332:u32)
      n275 = local read "framesPerSecond"() -> (w345:u32)
      n276 = Select(t=w332, s="fast forward", f=w329) -> (s? t:f=w324:u32)
      n277 = Subtract(x="Progress...", y=2) -> (x-y=w325:u32)
      n278 = Divide(x=1000.0, y=w340) -> (x/y=w344:dbl)
      n279 = Divide(x=w344, y=w345) -> (x/y=w342:dbl)
      n280 = Select(t=w325, s="fast rewind", f=w324) -> (s? t:f=w323:u32)
      n281 = Round Toward -Infinity(1:w342) -> (0:w341:dbl)
      "playback speed" <- w341
      n282 = Wait (ms)(milliseconds to wait=w341) -> ()  [unwired: 1 out]
      n283 = local read "Load video"() -> (w335:bool)
      n284 = Select(t="Progress...", s=w337, f=w323) -> (s? t:f=w336:u32)
      n285 = case shown="False" w335 {
        tunnel: w346 -> [w363 _]
        tunnel: w336 -> [w364 _]
        tunnel: [w364 w365] -> w350
        tunnel: [w363 w368] -> w347
        frame False {
        }
        frame True {
          n286 = local read "frames 2 play"() -> (w368:i64[])
          n287 = Array Max & Min(array=w368) -> (max index (indices)=w367:i32)  [unwired: 3 out]
          n288 = property on="Progress..." class="Slide (strict)"("Scale.Maximum"=w367) -> ()  [unwired: 2 in, 2 out]
          n289 = local write "Load video"(FALSE ("Play")) -> ()
          n290 = local read "Progress..."() -> (w365:u32)
        }
      }
      n291 = local write "Progress..."(w350) -> ()
      n292 = local read "START"() -> (w331:bool)
    }
    n293 = while {
      shift-right: [w372] -> _
      shift-left: T1."Display" ("Main tab") -> [w373]
      tunnel: w10 -> [w386]
      shift-right: [w376] -> _
      shift-left: w11 -> [w389]
      tunnel: w8 -> [_]
      tunnel: w1 -> [_]
      tunnel: [w374] -> w7
      stop <- w375 continue-if-true
      w379 = T1."Coding" ("Main tab")
      # "Moving to display tab"
      n294 = case shown="\"Edit video\"" w373 {
        tunnel: w389 -> [w548 w957 w1463 w1624 w1700 w1792]
        tunnel: [w420 w957 w1463 w1624 w1700 w1777] -> w376
        tunnel: [T1."Edit video" ("Main tab") w960 T1."Display" ("Main tab") T1."Edit coding" ("Main tab") w1701 T1."Edit video" ("Main tab")] -> w381
        tunnel: w386 -> [w435 _ _ _ _ _]
        tunnel: [w415 w952 w1461 w1622 w1698 w1775] -> w374
        frame "Coding", Default {
          w409 = "\t"
          w427 = "\r"
          n295 = local read "1 6"() -> (w531:bool)
          n296 = local read "2 6"() -> (w532:bool)
          n297 = local read "3 6"() -> (w533:bool)
          n298 = local read "4 6"() -> (w534:bool)
          n299 = local read "5 6"() -> (w535:bool)
          n300 = local read "6 6"() -> (w536:bool)
          n301 = local read "7 6"() -> (w538:bool)
          n302 = local read "8 6"() -> (w537:bool)
          n303 = local read "1 5"() -> (w539:bool)
          n304 = local read "2 5"() -> (w540:bool)
          n305 = local read "3 5"() -> (w541:bool)
          n306 = local read "4 5"() -> (w542:bool)
          n307 = local read "5 5"() -> (w543:bool)
          n308 = local read "6 5"() -> (w544:bool)
          n309 = local read "7 5"() -> (w545:bool)
          n310 = local read "8 5"() -> (w546:bool)
          n311 = Build Array(w531, w532, w533, w534, w535, w536, w538, w537, w539, w540, w541, w542, w543, w544, w545, w546) -> (w433:bool[])
          n312 = local read "1 4"() -> (w515:bool)
          n313 = local read "2 4"() -> (w516:bool)
          n314 = local read "3 4"() -> (w517:bool)
          n315 = local read "4 4"() -> (w518:bool)
          n316 = local read "5 4"() -> (w519:bool)
          n317 = local read "6 4"() -> (w520:bool)
          n318 = local read "7 4"() -> (w521:bool)
          n319 = local read "8 4"() -> (w522:bool)
          n320 = local read "1 3"() -> (w523:bool)
          n321 = local read "2 3"() -> (w524:bool)
          n322 = local read "3 3"() -> (w525:bool)
          n323 = local read "4 3"() -> (w526:bool)
          n324 = local read "5 3"() -> (w527:bool)
          n325 = local read "6 3"() -> (w528:bool)
          n326 = local read "7 3"() -> (w529:bool)
          n327 = local read "8 3"() -> (w530:bool)
          n328 = Build Array(w515, w516, w517, w518, w519, w520, w521, w522, w523, w524, w525, w526, w527, w528, w529, w530) -> (w432:bool[])
          n329 = local read "1 2"() -> (w499:bool)
          n330 = local read "2 2"() -> (w500:bool)
          n331 = local read "3 2"() -> (w501:bool)
          n332 = local read "4 2"() -> (w502:bool)
          n333 = local read "5 2"() -> (w503:bool)
          n334 = local read "6 2"() -> (w504:bool)
          n335 = local read "7 2"() -> (w505:bool)
          n336 = local read "8 2"() -> (w506:bool)
          n337 = local read "1"() -> (w507:bool)
          n338 = local read "2"() -> (w508:bool)
          n339 = local read "3"() -> (w509:bool)
          n340 = local read "4"() -> (w510:bool)
          n341 = local read "5"() -> (w511:bool)
          n342 = local read "6"() -> (w512:bool)
          n343 = local read "7"() -> (w513:bool)
          n344 = local read "8"() -> (w514:bool)
          n345 = Build Array(w499, w500, w501, w502, w503, w504, w505, w506, w507, w508, w509, w510, w511, w512, w513, w514) -> (w468:bool[])
          n346 = local read "MR  2"() -> (w497:bool)
          n347 = local read "MR  3"() -> (w498:bool)
          n348 = local read "MC 2"() -> (w495:bool)
          n349 = local read "MC 3"() -> (w496:bool)
          n350 = local read "BC 3"() -> (w483:bool)
          n351 = local read "BC 2"() -> (w484:bool)
          n352 = local read "TC 2"() -> (w489:bool)
          n353 = local read "TC 3"() -> (w490:bool)
          n354 = local read "ML 3"() -> (w493:bool)
          n355 = local read "ML 2"() -> (w494:bool)
          n356 = local read "BR 2"() -> (w485:bool)
          n357 = local read "BR 3"() -> (w486:bool)
          n358 = local read "TR 2"() -> (w491:bool)
          n359 = local read "TR 3"() -> (w492:bool)
          n360 = local read "BL 3"() -> (w481:bool)
          n361 = local read "BL 2"() -> (w482:bool)
          n362 = local read "TL 3"() -> (w487:bool)
          n363 = local read "TL 2"() -> (w488:bool)
          n364 = Build Array(w481, w482, w483, w484, w485, w486, w487, w488, w489, w490, w491, w492, w493, w494, w495, w496, w497, w498) -> (w431:bool[])
          n365 = local read "Player 1"() -> (w469:bool)
          n366 = local read "Player 2"() -> (w470:bool)
          n367 = local read "Pause"() -> (w407:bool)
          n368 = local read "Button 1"() -> (w406:bool)
          n369 = local read "Button 2"() -> (w405:bool)
          n370 = local read "Button 3"() -> (w404:bool)
          n371 = local read "Button 4"() -> (w403:bool)
          n372 = local read "Button 5"() -> (w402:bool)
          n373 = local read "W1"() -> (w471:bool)
          n374 = local read "W2"() -> (w472:bool)
          n375 = local read "1 7"() -> (w477:bool)
          n376 = local read "2 7"() -> (w478:bool)
          n377 = local read "3 7"() -> (w479:bool)
          n378 = local read "4 7"() -> (w480:bool)
          n379 = local read "E1"() -> (w473:bool)
          n380 = local read "E2"() -> (w474:bool)
          n381 = local read "S1"() -> (w475:bool)
          n382 = local read "S2"() -> (w476:bool)
          n383 = Build Array(w469, w470, w471, w472, w473, w474, w475, w476, w477, w478, w479, w480, w407, w406, w405, w404, w403, w402) -> (w430:bool[])
          n384 = Build Array(w433, w432, w468, w431, w430) -> (w466:bool[][])
          n385 = Or Array Elements(Boolean array=w466) -> (logical OR=w467:bool)
          n386 = control-ref of="Player 1"() -> (w436:refnum<vi>)
          n387 = control-ref of="Player 2"() -> (w437:refnum<vi>)
          n388 = control-ref of="E1"() -> (w438:refnum<vi>)
          n389 = control-ref of="E2"() -> (w439:refnum<vi>)
          n390 = control-ref of="W1"() -> (w440:refnum<vi>)
          n391 = control-ref of="W2"() -> (w441:refnum<vi>)
          n392 = control-ref of="S2"() -> (w442:refnum<vi>)
          n393 = control-ref of="S1"() -> (w443:refnum<vi>)
          n394 = control-ref of="TL 3"() -> (w444:refnum<vi>)
          n395 = control-ref of="TL 2"() -> (w445:refnum<vi>)
          n396 = control-ref of="TC 3"() -> (w446:refnum<vi>)
          n397 = control-ref of="TC 2"() -> (w447:refnum<vi>)
          n398 = control-ref of="TR 3"() -> (w448:refnum<vi>)
          n399 = control-ref of="TR 2"() -> (w449:refnum<vi>)
          n400 = control-ref of="ML 3"() -> (w450:refnum<vi>)
          n401 = control-ref of="ML 2"() -> (w451:refnum<vi>)
          n402 = control-ref of="MC 3"() -> (w452:refnum<vi>)
          n403 = control-ref of="MC 2"() -> (w453:refnum<vi>)
          n404 = control-ref of="MR  3"() -> (w454:refnum<vi>)
          n405 = control-ref of="MR  2"() -> (w455:refnum<vi>)
          n406 = control-ref of="BL 3"() -> (w456:refnum<vi>)
          n407 = control-ref of="BL 2"() -> (w457:refnum<vi>)
          n408 = control-ref of="BC 3"() -> (w458:refnum<vi>)
          n409 = control-ref of="BC 2"() -> (w459:refnum<vi>)
          n410 = control-ref of="BR 3"() -> (w460:refnum<vi>)
          n411 = control-ref of="BR 2"() -> (w461:refnum<vi>)
          n412 = local read "Video Frame"() -> (w434:u32)
          n413 = Build Array(w436, w437, w438, w439, w440, w441, w442, w443, w444, w445, w446, w447, w448, w449, w450, w451, w452, w453, w454, w455, w456, w457, w458, w459, w460, w461) -> (w464:refnum<vi>[])
          n414 = Array Size(array=w464) -> (size(s)=w462:i32)
          n415 = Divide(x=w462, y=2) -> (x/y=w465:dbl)
          n416 = case shown="True" w467 {
            tunnel: w434 -> [_ w581]
            tunnel: w548 -> [w564 w582]
            tunnel: [w564 w570] -> w420
            tunnel: w435 -> [_ w572]
            frame False {
            }
            frame True {
              n417 = stacked-sequence {
                tunnel: [_ _ w683 _ _ _ _ _ _] -> w587
                tunnel: [_ _ w682 _ _ _ _ _ _] -> w624
                tunnel: [_ _ w681 _ _ _ _ _ _] -> w623
                tunnel: [_ _ w680 _ _ _ _ _ _] -> w622
                tunnel: [_ _ w679 _ _ _ _ _ _] -> w621
                tunnel: [_ _ w678 _ _ _ _ _ _] -> w620
                tunnel: [_ _ w677 _ _ _ _ _ _] -> w619
                tunnel: [_ _ w676 _ _ _ _ _ _] -> w613
                tunnel: [_ _ w675 _ _ _ _ _ _] -> w618
                tunnel: [_ _ _ w714 _ _ _ _ _] -> w617
                tunnel: [_ _ _ w713 _ _ _ _ _] -> w616
                tunnel: [_ _ _ w711 _ _ _ _ _] -> w615
                tunnel: [_ _ _ _ w821 _ _ _ _] -> w614
                tunnel: [_ _ _ _ w818 _ _ _ _] -> w612
                tunnel: [_ _ _ _ w785 _ _ _ _] -> w611
                tunnel: [_ _ _ _ w784 _ _ _ _] -> w610
                tunnel: [_ _ _ _ w783 _ _ _ _] -> w609
                tunnel: [_ _ _ _ w782 _ _ _ _] -> w608
                tunnel: [_ _ _ _ w781 _ _ _ _] -> w607
                tunnel: [_ _ _ _ w780 _ _ _ _] -> w606
                tunnel: [_ _ _ _ w779 _ _ _ _] -> w605
                tunnel: [_ _ _ _ w778 _ _ _ _] -> w604
                tunnel: [_ _ _ _ _ _ _ w887 _] -> w603
                tunnel: [_ _ _ _ _ _ _ w886 _] -> w602
                tunnel: [_ _ _ _ _ _ _ w885 _] -> w601
                tunnel: [_ _ _ _ _ _ _ w884 _] -> w600
                tunnel: [_ _ _ _ _ _ _ w883 _] -> w599
                tunnel: [_ _ _ _ _ _ _ w882 _] -> w598
                tunnel: [_ _ _ _ _ _ w861 _ _] -> w597
                tunnel: [_ _ _ _ _ _ w861 _ _] -> w596
                tunnel: [_ _ _ _ _ _ w867 _ _] -> w595
                tunnel: [_ _ _ _ _ _ w866 _ _] -> w594
                tunnel: [_ _ _ _ _ _ w865 _ _] -> w593
                tunnel: [_ _ _ _ _ _ w864 _ _] -> w592
                tunnel: [_ _ _ _ _ _ w863 _ _] -> w591
                tunnel: [_ _ _ _ _ _ w862 _ _] -> w590
                tunnel: [_ _ _ _ _ w831 _ _ _] -> w589
                tunnel: [_ _ _ _ _ w829 _ _ _] -> w588
                tunnel: w582 -> [_ _ _ _ _ _ _ w881 _]
                tunnel: [_ _ _ _ _ _ _ w879 _] -> w577
                tunnel: w581 -> [w634 _ _ _ _ _ _ w880 _]
                tunnel: [w634 _ _ _ _ _ _ _ _] -> w580
                tunnel: w572 -> [w633 _ _ _ _ _ _ _ _]
                tunnel: [w628 _ _ _ _ _ _ _ _] -> w571
                tunnel: [_ _ _ _ w777 _ _ _ _] -> w569
                tunnel: [_ _ _ _ w771 _ _ _ _] -> w568
                tunnel: [_ _ _ _ w770 _ _ _ _] -> w567
                tunnel: [_ _ _ _ w769 _ _ _ _] -> w566
                tunnel: [_ _ _ _ w768 _ _ _ _] -> w565
                frame #0 {
                  n418 = local read "Pause"() -> (w631:bool)
                  n419 = Tick Count (ms)() -> (millisecond timer value=w629:u32)
                  n420 = And(x=w631, y="Pause lag on") -> (x .and. y?=w632:bool)
                  n421 = case shown="True" w632 {
                    tunnel: w634 -> [_ w651]
                    tunnel: w633 -> [_ w653]
                    tunnel: ["pauselag" ("Image Name") w649] -> w628
                    frame False {
                    }
                    frame True {
                      w654 = T5 4 items=["Grayscale (U8)", "Grayscale (I16)", "Grayscale (SGL)", "Complex (CSG)", "RGB (U32)", "HSL (U32)", "RGB (U64)"] ("Image Type")
                      n422 = local read "framesPerSecond"() -> (w660:u32)
                      n423 = local read "Number of Frames"() -> (w650:u32)
                      n424 = Increment(x=w651) -> (x+1=w652:u32)
                      n425 = Multiply(x="Pause lag(s)", y=w660) -> (x*y=w658:dbl)
                      n426 = call "IMAQ Create"("Image Name"="pauselag", "Image Type"=w654) -> ("New Image"=w649:T2, "error out"=w655:errorcluster)  [unwired: 3 in]
                      n427 = Round Toward +Infinity(x=w658) -> (ceil(x): smallest int >= x=w657:dbl)
                      n428 = for {
                        N: w657 -> [_]
                        tunnel: w652 -> [w667]
                        tunnel: w655 -> [w670]
                        tunnel: w649 -> [w669]
                        tunnel: w653 -> [w666]
                        tunnel: w650 -> [w664]
                        i -> [w668]
                        n429 = Add(x=w668, y=w667) -> (x+y=w663:u32)
                        n430 = local read "playback speed"() -> (w661:dbl)
                        n431 = Less Or Equal?(x=w664, y=w663) -> (x <= y?=w665:bool)
                        n432 = Select(t=w664, s=w665, f=w663) -> (s? t:f=w662:u32)
                        n433 = call "IMAQ AVI Read Frame"("error in (no error)"=w670, "Frame Number"=w662, "Image"=w669, "Avi Refnum"=w666) -> ("Image Out"=w671:T2)  [unwired: 4 in, 3 out]
                        n434 = local write "Video"(w671) -> ()
                        n435 = Wait (ms)(milliseconds to wait=w661) -> ()  [unwired: 1 out]
                      }
                    }
                  }
                  n436 = while {
                    tunnel: w629 -> [w646]
                    i -> [w637]
                    stop <- w644 stop-if-true
                    w640 = u32 25 ("milliseconds to wait")
                    n437 = Tick Count (ms)() -> (millisecond timer value=w647:u32)
                    n438 = Subtract(x=w647, y=w646) -> (x-y=w645:u32)
                    n439 = Multiply(x="Code lag(s)", y=1000) -> (x*y=w641:dbl)
                    n440 = Greater Or Equal?(x=w645, y=w641) -> (x >= y?=w644:bool)
                    n441 = Divide(x=w641, y=w640) -> (x/y=w639:dbl)
                    n442 = Divide(x=300.0, y=w639) -> (x/y=w636:dbl)
                    n443 = Multiply(x=w637, y=w636) -> (x*y=→"task":dbl)
                    n444 = Wait (ms)(milliseconds to wait=w640) -> ()  [unwired: 1 out]
                  }
                }
                frame #1 {
                  n445 = while {
                    stop <- w672 continue-if-true
                    n446 = local read "START"() -> (w673:bool)
                    n447 = local read "Pause"() -> (w674:bool)
                    n448 = And(x=w673, y=w674) -> (x .and. y?=w672:bool)
                  }
                }
                frame #2 {
                  n449 = Or(x="BC 3", y="BC 2") -> (x .or. y?=w685:bool)
                  n450 = Or(x="TC 2", y="TC 3") -> (x .or. y?=w691:bool)
                  n451 = Or(x="ML 3", y="ML 2") -> (x .or. y?=w689:bool)
                  n452 = Or(x="MR  2", y="MR  3") -> (x .or. y?=w687:bool)
                  n453 = Boolean To (0,1)(Boolean=w691) -> (0, 1=w682:i16)
                  n454 = Boolean To (0,1)(Boolean=w689) -> (0, 1=w680:i16)
                  n455 = Boolean To (0,1)(Boolean=w687) -> (0, 1=w678:i16)
                  n456 = Boolean To (0,1)(Boolean=w685) -> (0, 1=w676:i16)
                  n457 = Or(x="TL 3", y="TL 2") -> (x .or. y?=w692:bool)
                  n458 = Or(x="TR 2", y="TR 3") -> (x .or. y?=w690:bool)
                  n459 = Or(x="MC 2", y="MC 3") -> (x .or. y?=w688:bool)
                  n460 = Or(x="BL 3", y="BL 2") -> (x .or. y?=w686:bool)
                  n461 = Or(x="BR 2", y="BR 3") -> (x .or. y?=w684:bool)
                  n462 = Boolean To (0,1)(Boolean=w692) -> (0, 1=w683:i16)
                  n463 = Boolean To (0,1)(Boolean=w690) -> (0, 1=w681:i16)
                  n464 = Boolean To (0,1)(Boolean=w688) -> (0, 1=w679:i16)
                  n465 = Boolean To (0,1)(Boolean=w686) -> (0, 1=w677:i16)
                  n466 = Boolean To (0,1)(Boolean=w684) -> (0, 1=w675:i16)
                }
                frame #3 {
                  n467 = Build Array("1", "2", "3", "4", "5", "6", "7", "8", "1 2", "2 2", "3 2", "4 2", "5 2", "6 2", "7 2", "8 2") -> (w735:bool[])
                  "FH" <- w735
                  n468 = Or Array Elements(Boolean array=w735) -> (logical OR=w716:bool)
                  n469 = Boolean To (0,1)(Boolean=w716) -> (0, 1=w714:i16)
                  n470 = Build Array("1 3", "2 3", "3 3", "4 3", "5 3", "6 3", "7 3", "8 3", "1 4", "2 4", "3 4", "4 4", "5 4", "6 4", "7 4", "8 4") -> (w718:bool[])
                  "BH" <- w718
                  n471 = Or Array Elements(Boolean array=w718) -> (logical OR=w715:bool)
                  n472 = Boolean To (0,1)(Boolean=w715) -> (0, 1=w713:i16)
                  n473 = Build Array("1 5", "2 5", "3 5", "4 5", "5 5", "6 5", "7 5", "8 5", "1 6", "2 6", "3 6", "4 6", "5 6", "6 6", "7 6", "8 6") -> (w717:bool[])
                  "OH" <- w717
                  n474 = Or Array Elements(Boolean array=w717) -> (logical OR=w712:bool)
                  n475 = Boolean To (0,1)(Boolean=w712) -> (0, 1=w711:i16)
                }
                frame #4 {
                  w826 = 8 ("index")
                  n476 = local read "OH"() -> (w815:bool[])
                  n477 = local read "BH"() -> (w816:bool[])
                  n478 = local read "FH"() -> (w817:bool[])
                  n479 = Split 1D Array(array=w817, index=w826) -> (first subarray=w813:bool[], second subarray=w814:bool[])
                  n480 = Split 1D Array(array=w816, index=w826) -> (first subarray=w825:bool[], second subarray=w823:bool[])
                  n481 = Split 1D Array(array=w815, index=w826) -> (first subarray=w824:bool[], second subarray=w822:bool[])
                  n482 = Build Array(w813, w825, w824) -> (w812:bool[][])
                  n483 = Build Array(w814, w823, w822) -> (w811:bool[][])
                  n484 = Or Array Elements(Boolean array=w812) -> (logical OR=w820:bool)
                  n485 = Or Array Elements(Boolean array=w811) -> (logical OR=w819:bool)
                  n486 = Insert Into Array(array=w812, new element=w811) -> (w810:bool[][])  [unwired: 2 in]
                  n487 = Boolean To (0,1)(Boolean=w820) -> (0, 1=w821:i16)
                  n488 = Boolean To (0,1)(Boolean=w819) -> (0, 1=w818:i16)
                  n489 = Index Array(array=w810, index (col) #1=3 ("disabled index (col)"), index (col) #2=4 ("index (col)"), index (col) #3=2 ("index (col)"), index (col) #4=1 ("index (col)"), index (col) #5=6 ("index (col)"), index (col) #6=5 ("index (col)"), index (col) #7=0 ("index (col)"), index (col) #8=7 ("index (col)")) -> (element #1=w800:bool[], element #2=w792:bool[], element #3=w791:bool[], element #4=w790:bool[], element #5=w789:bool[], element #6=w788:bool[], element #7=w787:bool[], element #8=w786:bool[])  [unwired: 8 in]
                  n490 = Or Array Elements(Boolean array=w800) -> (logical OR=w801:bool)
                  n491 = Or Array Elements(Boolean array=w791) -> (logical OR=w797:bool)
                  n492 = Or Array Elements(Boolean array=w789) -> (logical OR=w796:bool)
                  n493 = Or Array Elements(Boolean array=w787) -> (logical OR=w793:bool)
                  n494 = Or Array Elements(Boolean array=w792) -> (logical OR=w799:bool)
                  n495 = Or Array Elements(Boolean array=w790) -> (logical OR=w798:bool)
                  n496 = Or Array Elements(Boolean array=w788) -> (logical OR=w795:bool)
                  n497 = Or Array Elements(Boolean array=w786) -> (logical OR=w794:bool)
                  n498 = Boolean To (0,1)(Boolean=w801) -> (0, 1=w785:i16)
                  n499 = Boolean To (0,1)(Boolean=w797) -> (0, 1=w783:i16)
                  n500 = Boolean To (0,1)(Boolean=w796) -> (0, 1=w781:i16)
                  n501 = Boolean To (0,1)(Boolean=w793) -> (0, 1=w779:i16)
                  n502 = Boolean To (0,1)(Boolean=w799) -> (0, 1=w784:i16)
                  n503 = Boolean To (0,1)(Boolean=w798) -> (0, 1=w782:i16)
                  n504 = Boolean To (0,1)(Boolean=w795) -> (0, 1=w780:i16)
                  n505 = Boolean To (0,1)(Boolean=w794) -> (0, 1=w778:i16)
                  n506 = Boolean To (0,1)(Boolean="Button 1") -> (0, 1=w777:i16)
                  n507 = Boolean To (0,1)(Boolean="Button 2") -> (0, 1=w771:i16)
                  n508 = Boolean To (0,1)(Boolean="Button 3") -> (0, 1=w770:i16)
                  n509 = Boolean To (0,1)(Boolean="Button 4") -> (0, 1=w769:i16)
                  n510 = Boolean To (0,1)(Boolean="Button 5") -> (0, 1=w768:i16)
                }
                frame #5 {
                  w836 = i16 1 ("t")
                  n511 = local read "S1"() -> (w828:bool)
                  n512 = local read "S2"() -> (w827:bool)
                  n513 = local read "MR  3"() -> (w852:bool)
                  n514 = local read "MC 3"() -> (w856:bool)
                  n515 = local read "TC 3"() -> (w857:bool)
                  n516 = local read "BC 3"() -> (w855:bool)
                  n517 = local read "ML 3"() -> (w858:bool)
                  n518 = local read "BR 3"() -> (w854:bool)
                  n519 = local read "TR 3"() -> (w853:bool)
                  n520 = local read "BL 3"() -> (w860:bool)
                  n521 = local read "TL 3"() -> (w859:bool)
                  n522 = Compound Arithmetic op=OR(w860, w859, w858, w857, w856, w855, w854, w853, w852) -> (w841:bool)
                  "P1 position" <- w841
                  n523 = local read "MR  2"() -> (w846:bool)
                  n524 = local read "MC 2"() -> (w848:bool)
                  n525 = local read "TC 2"() -> (w849:bool)
                  n526 = local read "BC 2"() -> (w847:bool)
                  n527 = local read "ML 2"() -> (w843:bool)
                  n528 = local read "TR 2"() -> (w845:bool)
                  n529 = local read "BR 2"() -> (w844:bool)
                  n530 = local read "BL 2"() -> (w851:bool)
                  n531 = local read "TL 2"() -> (w850:bool)
                  n532 = Compound Arithmetic op=OR(w851, w850, w843, w849, w848, w847, w846, w845, w844) -> (w839:bool)
                  "P2 position" <- w839
                  n533 = Compound Arithmetic op=OR(w841, "Player 1", w828) -> (w842:bool)
                  n534 = Compound Arithmetic op=OR(w839, "Player 2", w827) -> (w838:bool)
                  n535 = Boolean To (0,1)(Boolean=w842) -> (0, 1=w832:i16)
                  n536 = Boolean To (0,1)(Boolean=w838) -> (0, 1=w830:i16)
                  n537 = Equal To 0?(x=w830) -> (x = 0?=w834:bool)
                  n538 = Equal To 0?(x=w832) -> (x = 0?=w833:bool)
                  n539 = And(x=w833, y=w834) -> (x .and. y?=w835:bool)
                  n540 = Select(t=w836, s=w835, f=w832) -> (s? t:f=w831:i16)
                  n541 = Select(t=w836, s=w835, f=w830) -> (s? t:f=w829:i16)
                }
                frame #6 {
                  w861 = i16 0
                  n542 = Boolean To (0,1)(Boolean="S1") -> (0, 1=w867:i16)
                  n543 = Boolean To (0,1)(Boolean="S2") -> (0, 1=w866:i16)
                  n544 = Boolean To (0,1)(Boolean="1 7") -> (0, 1=w865:i16)
                  n545 = Boolean To (0,1)(Boolean="2 7") -> (0, 1=w864:i16)
                  n546 = Boolean To (0,1)(Boolean="3 7") -> (0, 1=w863:i16)
                  n547 = Boolean To (0,1)(Boolean="4 7") -> (0, 1=w862:i16)
                }
                frame #7 {
                  n548 = local read "P1 position"() -> (w894:bool)
                  n549 = local read "OH"() -> (w895:bool[])
                  n550 = local read "FH"() -> (w897:bool[])
                  n551 = local read "Button 1"() -> (w874:bool)
                  n552 = local read "Button 2"() -> (w875:bool)
                  n553 = local read "Button 3"() -> (w876:bool)
                  n554 = local read "Button 4"() -> (w877:bool)
                  n555 = local read "Button 5"() -> (w878:bool)
                  n556 = local read "S1"() -> (w900:bool)
                  n557 = local read "S2"() -> (w901:bool)
                  n558 = local read "BH"() -> (w896:bool[])
                  n559 = local read "P2 position"() -> (w890:bool)
                  n560 = Or Array Elements(Boolean array=w897) -> (logical OR=w893:bool)
                  n561 = Or Array Elements(Boolean array=w895) -> (logical OR=w891:bool)
                  n562 = Not(x="Link Errors") -> (.not. x?=w906:bool)
                  n563 = local read "Player 1"() -> (w898:bool)
                  n564 = local read "Player 2"() -> (w899:bool)
                  n565 = Or Array Elements(Boolean array=w896) -> (logical OR=w892:bool)
                  n566 = local read "1 7"() -> (w902:bool)
                  n567 = local read "2 7"() -> (w903:bool)
                  n568 = local read "3 7"() -> (w904:bool)
                  n569 = local read "4 7"() -> (w905:bool)
                  n570 = Compound Arithmetic op=OR(w906, w894, w893, w892, w891, w890, w898, w899, w900, w901, w902, w903, w904, w905, w874, w875, w876, w877, w878) -> (w888:bool)
                  n571 = case shown="False" w888 {
                    tunnel: [w907 w947] -> w887
                    tunnel: [w907 w946] -> w886
                    tunnel: [w907 w945] -> w885
                    tunnel: [w907 w944] -> w884
                    tunnel: [w907 w943] -> w883
                    tunnel: [w907 w942] -> w882
                    tunnel: w881 -> [w911 w941]
                    tunnel: w880 -> [w930 _]
                    tunnel: [w910 w941] -> w879
                    frame False {
                      w907 = i16 0
                      n572 = local read "W1"() -> (w926:bool)
                      n573 = local read "W2"() -> (w927:bool)
                      n574 = local read "E1"() -> (w928:bool)
                      n575 = local read "E2"() -> (w929:bool)
                      n576 = Index Array(array=w911, index (col)=0 ("disabled index (col)")) -> (element=w931:i64[])  [unwired: 1 in]
                      n577 = for {
                        tunnel: w931 -> [w934] mode=indexing
                        tunnel: w930 -> [w935]
                        tunnel: [w934] -> w933 mode=indexing if=w936
                        stop <- w936 continue-if-true
                        n578 = Less Or Equal?(x=w934, y=w935) -> (x <= y?=w936:bool)
                      }
                      n579 = Or(x=w926, y=w929) -> (x .or. y?=w925:bool)
                      n580 = Or(x=w927, y=w928) -> (x .or. y?=w924:bool)
                      n581 = Boolean To (0,1)(Boolean=w926) -> (0, 1=w921:i16)
                      n582 = Boolean To (0,1)(Boolean=w927) -> (0, 1=w920:i16)
                      n583 = Boolean To (0,1)(Boolean=w928) -> (0, 1=w915:i16)
                      n584 = Boolean To (0,1)(Boolean=w929) -> (0, 1=w914:i16)
                      n585 = Boolean To (0,1)(Boolean=w925) -> (0, 1=w913:i16)
                      n586 = Boolean To (0,1)(Boolean=w924) -> (0, 1=w912:i16)
                      n587 = Array Size(array=w933) -> (size(s)=w909:i32)
                      n588 = Decrement(x=w909) -> (x-1=w908:i32)
                      n589 = Replace Array Subset(array=w911, new element #1=w921, index (row) #1=w908, index (col) #1=23 ("disabled index (col)"), new element #2=w920, index (row) #2=w908, index (col) #2=24 ("disabled index (col)"), new element #3=w915, index (row) #3=w908, index (col) #3=25 ("disabled index (col)"), new element #4=w914, index (row) #4=w908, index (col) #4=26 ("disabled index (col)"), new element #5=w913, index (row) #5=w908, index (col) #5=27 ("disabled index (col)"), new element #6=w912, index (row) #6=w908, index (col) #6=28 ("disabled index (col)")) -> (w910:i64[][])
                    }
                    frame True {
                      n590 = Or(x="W1", y="E2") -> (x .or. y?=w948:bool)
                      n591 = Or(x="E1", y="W2") -> (x .or. y?=w949:bool)
                      n592 = Boolean To (0,1)(Boolean="W1") -> (0, 1=w947:i16)
                      n593 = Boolean To (0,1)(Boolean="E1") -> (0, 1=w946:i16)
                      n594 = Boolean To (0,1)(Boolean="W2") -> (0, 1=w945:i16)
                      n595 = Boolean To (0,1)(Boolean="E2") -> (0, 1=w944:i16)
                      n596 = Boolean To (0,1)(Boolean=w948) -> (0, 1=w943:i16)
                      n597 = Boolean To (0,1)(Boolean=w949) -> (0, 1=w942:i16)
                    }
                  }
                }
                frame #8 {
                  w950 = FALSE ("4 6")
                  n598 = local write "1 6"(w950) -> ()
                  n599 = local write "2 6"(w950) -> ()
                  n600 = local write "3 6"(w950) -> ()
                  n601 = local write "4 6"(w950) -> ()
                  n602 = local write "5 6"(w950) -> ()
                  n603 = local write "6 6"(w950) -> ()
                  n604 = local write "7 6"(w950) -> ()
                  n605 = local write "8 6"(w950) -> ()
                  n606 = local write "Player 1"(w950) -> ()
                  n607 = local write "Player 2"(w950) -> ()
                  n608 = local write "Button 1"(w950) -> ()
                  n609 = local write "Button 2"(w950) -> ()
                  n610 = local write "Button 3"(w950) -> ()
                  n611 = local write "Button 4"(w950) -> ()
                  n612 = local write "Button 5"(w950) -> ()
                  n613 = local write "1 5"(w950) -> ()
                  n614 = local write "2 5"(w950) -> ()
                  n615 = local write "3 5"(w950) -> ()
                  n616 = local write "4 5"(w950) -> ()
                  n617 = local write "5 5"(w950) -> ()
                  n618 = local write "6 5"(w950) -> ()
                  n619 = local write "7 5"(w950) -> ()
                  n620 = local write "8 5"(w950) -> ()
                  n621 = local write "1 4"(w950) -> ()
                  n622 = local write "2 4"(w950) -> ()
                  n623 = local write "3 4"(w950) -> ()
                  n624 = local write "4 4"(w950) -> ()
                  n625 = local write "5 4"(w950) -> ()
                  n626 = local write "6 4"(w950) -> ()
                  n627 = local write "7 4"(w950) -> ()
                  n628 = local write "8 4"(w950) -> ()
                  n629 = local write "1 3"(w950) -> ()
                  n630 = local write "2 3"(w950) -> ()
                  n631 = local write "3 3"(w950) -> ()
                  n632 = local write "4 3"(w950) -> ()
                  n633 = local write "5 3"(w950) -> ()
                  n634 = local write "6 3"(w950) -> ()
                  n635 = local write "7 3"(w950) -> ()
                  n636 = local write "8 3"(w950) -> ()
                  n637 = local write "1 2"(w950) -> ()
                  n638 = local write "2 2"(w950) -> ()
                  n639 = local write "3 2"(w950) -> ()
                  n640 = local write "4 2"(w950) -> ()
                  n641 = local write "5 2"(w950) -> ()
                  n642 = local write "6 2"(w950) -> ()
                  n643 = local write "7 2"(w950) -> ()
                  n644 = local write "8 2"(w950) -> ()
                  n645 = local write "1"(w950) -> ()
                  n646 = local write "2"(w950) -> ()
                  n647 = local write "3"(w950) -> ()
                  n648 = local write "4"(w950) -> ()
                  n649 = local write "5"(w950) -> ()
                  n650 = local write "6"(w950) -> ()
                  n651 = local write "7"(w950) -> ()
                  n652 = local write "8"(w950) -> ()
                  n653 = local write "BL 3"(w950) -> ()
                  n654 = local write "BL 2"(w950) -> ()
                  n655 = local write "BR 2"(w950) -> ()
                  n656 = local write "BR 3"(w950) -> ()
                  n657 = local write "BC 3"(w950) -> ()
                  n658 = local write "BC 2"(w950) -> ()
                  n659 = local write "W1"(w950) -> ()
                  n660 = local write "W2"(w950) -> ()
                  n661 = local write "E1"(w950) -> ()
                  n662 = local write "E2"(w950) -> ()
                  n663 = local write "1 7"(w950) -> ()
                  n664 = local write "2 7"(w950) -> ()
                  n665 = local write "3 7"(w950) -> ()
                  n666 = local write "4 7"(w950) -> ()
                  n667 = local write "TL 3"(w950) -> ()
                  n668 = local write "TL 2"(w950) -> ()
                  n669 = local write "TR 2"(w950) -> ()
                  n670 = local write "TR 3"(w950) -> ()
                  n671 = local write "TC 2"(w950) -> ()
                  n672 = local write "TC 3"(w950) -> ()
                  n673 = local write "S1"(w950) -> ()
                  n674 = local write "S2"(w950) -> ()
                  n675 = local write "ML 3"(w950) -> ()
                  n676 = local write "ML 2"(w950) -> ()
                  n677 = local write "MR  2"(w950) -> ()
                  n678 = local write "MR  3"(w950) -> ()
                  n679 = local write "MC 2"(w950) -> ()
                  n680 = local write "MC 3"(w950) -> ()
                }
              }
              n681 = Build Array(w580, w587, w624, w623, w622, w621, w620, w619, w613, w618, w617, w616, w615, w614, w612, w611, w610, w609, w608, w607, w606, w605, w604, w603, w602, w601, w600, w599, w598, w597, w596, w595, w594, w593, w592, w591, w590, w589, w588, w569, w568, w567, w566, w565) -> (w576:u32[])
              n682 = call "IMAQ Dispose"("Image"=w571) -> ()  [unwired: 5 in, 1 out]
              n683 = Index Array(array=w577, index (col)=0 ("disabled index (col)")) -> (element=w586:i64[])  [unwired: 1 in]
              n684 = Delete From Array(array=w576, index=0) -> (array with subset deleted=w578:u32[])  [unwired: 1 in, 1 out]
              n685 = for {
                tunnel: w586 -> [w625] mode=indexing
                tunnel: w580 -> [w626]
                tunnel: [w625] -> w584 mode=indexing if=w627
                stop <- w627 continue-if-true
                n686 = Less Or Equal?(x=w625, y=w626) -> (x <= y?=w627:bool)
              }
              n687 = Array Max & Min(array=w578) -> (max value=w575:u32)  [unwired: 3 out]
              n688 = Equal To 0?(x=w575) -> (x = 0?=w573:bool)
              n689 = Array Size(array=w584) -> (size(s)=w583:i32)
              n690 = Insert Into Array(array=w577, index (row)=w583, new element=w576) -> (w574:i64[][])  [unwired: 1 in]
              n691 = Select(t=w577, s=w573, f=w574) -> (s? t:f=w570:i64[][])
            }
          }
          n692 = case shown="True" "Switch position" {
            tunnel: w464 -> [_ w551]
            tunnel: w465 -> [_ w550]
            frame False {
            }
            frame True {
              n693 = for {
                N: w550 -> [_]
                tunnel: w551 -> [w558]
                i -> [w557]
                n694 = Multiply(x=2, y=w557) -> (x*y=w555:i32)
                n695 = Increment(x=w555) -> (x+1=w554:i32)
                n696 = Index Array(array=w558, index #1=w555, index #2=w554) -> (element #1=w552:refnum<vi>, element #2=w553:refnum<vi>)
                n697 = property class="Bool (strict)"(reference=w552) -> (error out=w563:errorcluster, "Position"=w560:T8)  [unwired: 1 in, 1 out]
                n698 = property class="Bool (strict)"(reference=w553, error in=w563) -> (error out=w562:errorcluster, "Position"=w559:T8)  [unwired: 1 out]
                n699 = property class="Bool (strict)"(reference=w553, error in=w562, "Position"=w560) -> (error out=w561:errorcluster)  [unwired: 1 out]
                n700 = property class="Bool (strict)"(reference=w552, error in=w561, "Position"=w559) -> ()  [unwired: 2 out]
              }
              n701 = local write "Switch position"(FALSE ("Switch position")) -> ()
            }
          }
          n702 = Concatenate Strings("Btn 1", w409, "Btn 2", w409, "Btn 3", w409, "Btn 4", w409, "Btn 5") -> (w408:string)
          n703 = call "EVENTS(SubVI).vi"("concatenated string"=w408) -> ("Events"=w425:string)
          n704 = local read "Video file"() -> (w423:path)
          n705 = local read "Data file"() -> (w416:path)
          n706 = call <vilib>:"Get File Extension.vi"("file"=w423) -> ("filename without extension"=w426:string)  [unwired: 7 in, 3 out]
          n707 = Array To Spreadsheet String(delimiter (Tab)="\t" ("delimiter (\\t)"), array=w420, 3:"%.3f" ("format (%.3f)")) -> (spreadsheet string=w429:string)
          n708 = Open/Create/Replace File(file path (use dialog)=w416, operation (0:open)=T3."replace") -> (refnum out=w418:refnum<file>, error out=w417:errorcluster)  [unwired: 4 in, 1 out]
          n709 = Concatenate Strings("avi file" ("string"), w427, w426, w427, w427, w425, w429) -> (w428:string)
          n710 = Write to Text File(file (use dialog)=w418, text=w428, error in=w417) -> (refnum out=w415:refnum<file>)  [unwired: 1 in, 2 out]
          "coding" <- w548
        }
        frame "Display" {
          n711 = stacked-sequence {
            tunnel: w957 -> [w1049 w1169]
            frame #0 {
              w1039 = i64 0 ("new element/subarray")
              w1038 = i64 0 ("new element/subarray")
              w1037 = i64 0 ("new element/subarray")
              w1009 = 0.0 ("disabled index (col)")
              n712 = Index Array(array=w1049, index (col) #1=31 ("length"), index (col) #2=32 ("disabled index (col)"), index (col) #3=27 ("index (col)"), index (col) #4=28 ("index (col)")) -> (element #1=w1029:i64[], element #2=w1030:i64[], element #3=w1008:i64[], element #4=w1007:i64[])  [unwired: 4 in]
              n713 = Index Array(array=w1049, index (col)=0 ("disabled index (col)")) -> (element=w972:i64[])  [unwired: 1 in]
              n714 = Or(x=w1008, y=w1007) -> (x .or. y?=w984:i64[])
              n715 = Or(x=w1029, y=w1030) -> (x .or. y?=w1031:i64[])
              n716 = for {
                shift-right: [w1083] -> _
                shift-left: w1009 -> [w1082]
                shift-right: [w1081] -> _
                shift-left: w1009 -> [w1080]
                tunnel: w1007 -> [w1086] mode=indexing
                tunnel: w1008 -> [w1093] mode=indexing
                tunnel: [w1077] -> w970 mode=indexing if=w1075
                tunnel: [w1076] -> w971 mode=indexing if=w1075
                w1085 = 1.0 ("x")
                w1090 = 1.0 ("x")
                n717 = Equal?(x=w1090, y=w1093) -> (x = y?=w1087:bool)
                n718 = Add(x=w1080, y=w1085) -> (x+y=w1084:dbl)
                n719 = Add(x=w1090, y=w1082) -> (x+y=w1089:dbl)
                n720 = Equal?(x=w1086, y=w1085) -> (x = y?=w1092:bool)
                n721 = Or(x=w1087, y=w1092) -> (x .or. y?=w1075:bool)
                n722 = Select(t=0.0, s=w1092, f=w1089) -> (s? t:f=w1078:dbl)
                n723 = Select(t=0.0, s=w1087, f=w1084) -> (s? t:f=w1076:dbl)
                n724 = Multiply(x=-1.0 ("y"), y=w1078) -> (x*y=w1077:dbl)
                n725 = Select(t=w1078, s=w1075, f=w1082) -> (s? t:f=w1083:dbl)
                n726 = Select(t=w1076, s=w1075, f=w1080) -> (s? t:f=w1081:dbl)
              }
              "p1y" <- w970
              "p2y" <- w971
              n727 = for {
                tunnel: w1031 -> [w1166] mode=indexing
                tunnel: w972 -> [w1163] mode=indexing
                tunnel: [w1163] -> w985 mode=indexing if=w1165
                tunnel: w984 -> [w1164] mode=indexing
                tunnel: [w1163] -> w983 mode=indexing if=w1162
                w1161 = 1.0 ("x")
                n728 = Equal?(x=w1161, y=w1166) -> (x = y?=w1165:bool)
                n729 = Equal?(x=w1161, y=w1164) -> (x = y?=w1162:bool)
              }
              "service frames" <- w985
              "point frames" <- w983
              n730 = for {
                tunnel: w1008 -> [w1151] mode=indexing
                tunnel: w1007 -> [w1147] mode=indexing
                shift-right: [w1143] -> _
                shift-left: dbl[] [] -> [w1146]
                shift-right: [w1141] -> w1044
                shift-left: dbl[][] [] -> [w1140]
                n731 = Index Array(array=w1146, index #1=0 ("index"), index #2=1 ("index")) -> (element #1=w1152:dbl, element #2=w1150:dbl)
                n732 = Add(x=w1151, y=w1152) -> (x+y=w1149:dbl)
                n733 = Add(x=w1150, y=w1147) -> (x+y=w1148:dbl)
                n734 = Build Array(w1149, w1148) -> (w1143:dbl[])
                n735 = Equal?(x=w1146, y=w1143) -> (x = y?=w1145:bool[])
                n736 = Insert Into Array(array=w1140, new element=w1143) -> (w1142:dbl[][])  [unwired: 2 in]
                n737 = And Array Elements(Boolean array=w1145) -> (logical AND=w1144:bool)
                n738 = Select(t=w1140, s=w1144, f=w1142) -> (s? t:f=w1141:dbl[][])
              }
              n739 = for {
                N -> [w1155]
                tunnel: w983 -> [w1160] mode=indexing
                tunnel: w985 -> [w1159] mode=indexing
                tunnel: [w1156] -> w1041 mode=indexing
                shift-right: [w1156] -> _
                shift-left: i64 0 -> [w1157]
                tunnel: [w1155] -> _ mode=indexing
                n740 = Subtract(x=w1160, y=w1159) -> (x-y=w1158:i64)
                n741 = Add(x=w1157, y=w1158) -> (x+y=w1156:i64)
              }
              n742 = Divide(x=w1041, y=i64 25 ("new element/subarray")) -> (x/y=w1040:dbl[])
              n743 = Index Array(array=w1049, index (col) #1=23 ("disabled index (col)"), index (col) #2=24 ("index (col)"), index (col) #3=25 ("index (col)"), index (col) #4=26 ("index (col)"), index (col) #5=0 ("index (col)")) -> (element #1=w1024:i64[], element #2=w978:i64[], element #3=w977:i64[], element #4=w976:i64[], element #5=w973:i64[])  [unwired: 5 in]
              n744 = Insert Into Array(array=w971, index=w1038, new element=w1038) -> (w1004:dbl[])
              n745 = Insert Into Array(array=w1040, index=w1037, new element=w1037) -> (w990:dbl[])
              n746 = Insert Into Array(array=w970, index=w1039, new element=w1039) -> (w1005:dbl[])
              n747 = Insert Into Array(array=w1044, index (row)=0, new element=dbl[] [0.0, 0.0] ("new element/subarray")) -> (w1003:dbl[][])  [unwired: 1 in]
              n748 = for {
                tunnel: w1024 -> [w1139] mode=indexing
                tunnel: w973 -> [w1137] mode=indexing
                tunnel: [w1137] -> w982 mode=indexing if=w1138
                tunnel: [w1137] -> w981 mode=indexing if=w1130
                tunnel: [w1137] -> w980 mode=indexing if=w1131
                tunnel: [w1137] -> w979 mode=indexing if=w1132
                tunnel: w978 -> [w1136] mode=indexing
                tunnel: w977 -> [w1135] mode=indexing
                tunnel: w976 -> [w1134] mode=indexing
                w1133 = 1 ("x")
                n749 = Equal?(x=w1133, y=w1139) -> (x = y?=w1138:bool)
                n750 = Equal?(x=w1133, y=w1136) -> (x = y?=w1130:bool)
                n751 = Equal?(x=w1133, y=w1135) -> (x = y?=w1131:bool)
                n752 = Equal?(x=w1133, y=w1134) -> (x = y?=w1132:bool)
              }
              n753 = property on="momentum graph" class="XYGraph (strict)"() -> ("Cursor.Cursor X"=w1047:dbl)  [unwired: 2 in, 2 out]
              n754 = Search 1D Array(1D array=w990, element=w1047) -> (index of element=w995:i32)  [unwired: 1 in]
              n755 = for {
                tunnel: w982 -> [w1129] mode=indexing
                tunnel: w983 -> [w1128]
                tunnel: [w1126] -> w1022 mode=indexing
                tunnel: [w1123] -> w1023 mode=indexing
                tunnel: w990 -> [w1122]
                tunnel: w1005 -> [w1121]
                n756 = Search 1D Array(1D array=w1128, element=w1129) -> (index of element=w1124:i32)  [unwired: 1 in]
                n757 = Increment(x=w1124) -> (x+1=w1127:i32)
                n758 = Increment(x=w1124) -> (x+1=w1125:i32)
                n759 = Index Array(array=w1122, index=w1127) -> (element=w1126:dbl)
                n760 = Index Array(array=w1121, index=w1125) -> (element=w1123:dbl)
              }
              n761 = for {
                tunnel: w980 -> [w1111] mode=indexing
                tunnel: w983 -> [w1110]
                tunnel: [w1108] -> w1017 mode=indexing
                tunnel: [w1105] -> w1016 mode=indexing
                tunnel: w990 -> [w1104]
                tunnel: w1004 -> [w1103]
                n762 = Search 1D Array(1D array=w1110, element=w1111) -> (index of element=w1106:i32)  [unwired: 1 in]
                n763 = Increment(x=w1106) -> (x+1=w1109:i32)
                n764 = Increment(x=w1106) -> (x+1=w1107:i32)
                n765 = Index Array(array=w1104, index=w1109) -> (element=w1108:dbl)
                n766 = Index Array(array=w1103, index=w1107) -> (element=w1105:dbl)
              }
              n767 = for {
                tunnel: w979 -> [w1102] mode=indexing
                tunnel: w983 -> [w1101]
                tunnel: [w1099] -> w1015 mode=indexing
                tunnel: [w1096] -> w1014 mode=indexing
                tunnel: w990 -> [w1095]
                tunnel: w1005 -> [w1094]
                n768 = Search 1D Array(1D array=w1101, element=w1102) -> (index of element=w1097:i32)  [unwired: 1 in]
                n769 = Increment(x=w1097) -> (x+1=w1100:i32)
                n770 = Increment(x=w1097) -> (x+1=w1098:i32)
                n771 = Index Array(array=w1095, index=w1100) -> (element=w1099:dbl)
                n772 = Index Array(array=w1094, index=w1098) -> (element=w1096:dbl)
              }
              n773 = for {
                tunnel: w981 -> [w1120] mode=indexing
                tunnel: w983 -> [w1119]
                tunnel: [w1117] -> w1025 mode=indexing
                tunnel: [w1114] -> w1026 mode=indexing
                tunnel: w990 -> [w1113]
                tunnel: w1004 -> [w1112]
                n774 = Search 1D Array(1D array=w1119, element=w1120) -> (index of element=w1115:i32)  [unwired: 1 in]
                n775 = Increment(x=w1115) -> (x+1=w1118:i32)
                n776 = Increment(x=w1115) -> (x+1=w1116:i32)
                n777 = Index Array(array=w1113, index=w1118) -> (element=w1117:dbl)
                n778 = Index Array(array=w1112, index=w1116) -> (element=w1114:dbl)
              }
              n779 = Decrement(x=w995) -> (x-1=w996:i32)
              n780 = Index Array(array=w1003, index (row)=w995) -> (element=→"Score":dbl[])  [unwired: 1 in]
              n781 = Array Max & Min(array=w990) -> (max value=w999:dbl)  [unwired: 3 out]
              n782 = Array Size(array=w1003) -> (size(s)=w1002:i32[])
              n783 = Index Array(array=w990, index #1=w995, index #2=w996) -> (element #1=w993:dbl, element #2=w994:dbl)
              n784 = Delete From Array(array=w990, index=0) -> (array with subset deleted=w989:dbl[])  [unwired: 1 in, 1 out]
              n785 = Index Array(array=w1002, index=0) -> (element=w1000:i32)
              n786 = Subtract(x=w993, y=w994) -> (x-y=→"Rally length(sec)":dbl)
              n787 = Subtract(x=w989, y=w990) -> (x-y=w988:dbl[])
              n788 = Decrement(x=w1000) -> (x-1=w998:i32)
              n789 = Array Max & Min(array=w988) -> (max value=→"Longest rally length(sec)":dbl, min value=→"Shortest rally length(sec)":dbl)  [unwired: 2 out]
              n790 = Bundle(w990, w1004) -> (w1034:cluster{dbl[], dbl[]})  [unwired: 1 in]
              n791 = Bundle(w1015, w1014) -> (w1010:cluster{dbl[], dbl[]})  [unwired: 1 in]
              n792 = Bundle(w990, w1005) -> (w1035:cluster{dbl[], dbl[]})  [unwired: 1 in]
              n793 = Bundle(w1025, w1026) -> (w1012:cluster{dbl[], dbl[]})  [unwired: 1 in]
              n794 = Bundle(w1017, w1016) -> (w1011:cluster{dbl[], dbl[]})  [unwired: 1 in]
              n795 = Bundle(w1022, w1023) -> (w1013:cluster{dbl[], dbl[]})  [unwired: 1 in]
              n796 = Divide(x=w999, y=w998) -> (x/y=→"Average rally length(sec)":dbl)
              n797 = Build Array(w1013, w1012, w1011, w1010, w1035, w1034) -> (→"momentum graph":cluster{dbl[], dbl[]}[])
              n798 = local read "Video files to write"() -> (w965:string[])
              n799 = property on="Video files to write" class="Arr (strict)"() -> ("Index Values"=w964:u32[])  [unwired: 2 in, 2 out]
              n800 = local read "frames to write"() -> (w966:i64[][])
              n801 = case shown="True" "Upload edited video" {
                frame False {
                }
                frame True {
                  n802 = flat-sequence {
                    frame #0 {
                      n803 = local read "frames edited"() -> (w1071:i64[])
                      n804 = local write "Progress..."(u32 0 ("Progress...")) -> ()
                      n805 = local write "frames 2 play"(w1071) -> ()
                    }
                    frame #1 {
                      w1073 = FALSE ("stop")
                      w1074 = TRUE ("Play")
                      n806 = local write "Load video"(w1074) -> ()
                      n807 = local write "Play"(w1074) -> ()
                      n808 = local write "stop"(w1073) -> ()
                      n809 = local write "Upload edited video"(w1073) -> ()
                      n810 = local write "Pause"(w1073) -> ()
                    }
                  }
                }
              }
              n811 = Index Array(array=w964) -> (element=w961:u32)  [unwired: 1 in]
              n812 = And Array Elements(Boolean array="Delete") -> (logical AND=w963:bool)
              n813 = case shown="True" "Add to lib" {
                tunnel: w966 -> [_ w1066]
                tunnel: w965 -> [_ w1063]
                frame False {
                }
                frame True {
                  n814 = local read "frames edited"() -> (w1062:i64[])
                  n815 = local write "Add to lib"(FALSE ("Add to lib")) -> ()
                  n816 = Build Array("File name") -> (w1064:string[])
                  n817 = Build Array(w1062) -> (w1067:i64[][])
                  n818 = Insert Into Array(array=w1067, new element=w1066) -> (→"frames to write":i64[][])  [unwired: 2 in]
                  n819 = Insert Into Array(array=w1064, new element=w1063) -> (→"Video files to write":string[])  [unwired: 1 in]
                }
              }
              n820 = case shown="False" w963 {
                tunnel: "Delete" -> [w1058 _]
                tunnel: w961 -> [w1056 _]
                frame False {
                  n821 = for {
                    tunnel: w1058 -> [w1061] mode=indexing
                    tunnel: [w1059] -> w1057
                    i -> [w1059]
                    stop <- w1060 stop-if-true
                    n822 = Not(x=w1061) -> (.not. x?=w1060:bool)
                  }
                  n823 = local write "Delete"(bool[] [TRUE, TRUE, TRUE, TRUE, TRUE] ("Array 2")) -> ()
                  n824 = local read "Video files to write"() -> (w1053:string[])
                  n825 = local read "frames to write"() -> (w1051:i64[][])
                  n826 = Add(x=w1057, y=w1056) -> (x+y=w1050:u32)
                  n827 = Delete From Array(array=w1053, index=w1050) -> (array with subset deleted=w1055:string[])  [unwired: 1 in, 1 out]
                  n828 = Delete From Array(array=w1051, index (row)=w1050) -> (array with subset deleted=w1052:i64[][])  [unwired: 2 in, 1 out]
                  n829 = local write "frames to write"(w1052) -> ()
                  n830 = local write "Video files to write"(w1055) -> ()
                }
                frame True {
                }
              }
            }
            frame #1 {
              w1209 = 0.0 ("X Scale.Range:Minimum")
              w1247 = i16 1 ("width (-)")
              w1385 = dbl[] [0.0, 0.0, 0.0, 0.0, 0.0, 0.0, 0.0, 0.0] ("array")
              w1371 = string[] ["Winners", "Errors"] ("W/E1")
              w1352 = string[] ["Fore hand", "Back hand", "Over head", "", "Straight", "Cross", "", "Smash", "Defence", "Drive/Tap", "Lob", "Drop", "Chop", "Clear", "Net"] ("Player 2")
              w1346 = "" ("new element/subarray")
              w1345 = "" ("new element/subarray")
              w1298 = 9 ("index")
              w1293 = 9 ("index")
              n831 = local read "edited\nevents"() -> (w1268:i64[][])
              n832 = local read "Compare"() -> (w1224:bool)
              n833 = case shown="\"4\"" "2 8" {
                tunnel: [w1392 w1393 w1394] -> w1256
                frame "1", Default {
                  n834 = local read "game"() -> (w1392:i32[][])
                }
                frame "3" {
                  n835 = local read "save1 2"() -> (w1393:i32[][])
                }
                frame "4" {
                  n836 = local read "save2 2"() -> (w1394:i32[][])
                }
              }
              n837 = case shown="\"3\"" "1 8" {
                tunnel: [w1395 w1396 w1397] -> w1260
                frame "1", Default {
                  n838 = local read "game"() -> (w1395:i32[][])
                }
                frame "3" {
                  n839 = local read "save1 2"() -> (w1396:i32[][])
                }
                frame "4" {
                  n840 = local read "save2 2"() -> (w1397:i32[][])
                }
              }
              n841 = case shown="False" w1224 {
                frame False {
                  w1386 = u8 0 ("Disabled")
                  n842 = local read "Percentage"() -> (w1387:bool)
                  n843 = local write "Percentage"(w1387) -> ()
                  n844 = local read "display\nselection"() -> (w1388:string)
                  n845 = local write "display\nselection"(w1388) -> ()
                  n846 = property on="display\nselection" class="CmbBox"("Disabled"=w1386) -> ()  [unwired: 2 in, 2 out]
                  n847 = property on="Percentage" class="Bool (strict)"("Disabled"=w1386) -> ()  [unwired: 2 in, 2 out]
                }
                frame True {
                  w1389 = u8 2 ("Disabled")
                  n848 = local read "1 8"() -> (w1391:string)
                  n849 = local write "display\nselection"(w1391) -> ()
                  n850 = property on="display\nselection" class="CmbBox"("Disabled"=w1389) -> ()  [unwired: 2 in, 2 out]
                  n851 = property on="Percentage" class="Bool (strict)"("Disabled"=w1389) -> ()  [unwired: 2 in, 2 out]
                  n852 = local write "Percentage"(TRUE ("t")) -> ()
                }
              }
              n853 = Index Array(array=w1169, index (col)=0 ("disabled index (col)")) -> (element=w1275:i64[])  [unwired: 1 in]
              n854 = Index Array(array=w1268, index (col)=0 ("disabled index (col)")) -> (element=w1273:i64[])  [unwired: 1 in]
              n855 = for {
                tunnel: w1275 -> [w1413]
                tunnel: w1273 -> [w1412] mode=indexing
                tunnel: [w1410] -> w1266 mode=indexing
                tunnel: w1169 -> [w1409]
                i -> [w1414]
                n856 = Search 1D Array(1D array=w1413, element=w1412, start index (0)=w1414) -> (index of element=w1411:i32)
                n857 = Index Array(array=w1409, index (row)=w1411) -> (element=w1410:i64[])  [unwired: 1 in]
              }
              n858 = Index Array(array=w1256, index (row) #1=0 ("index (row)"), index (row) #2=1 ("index (row)")) -> (element #1=w1254:i32[], element #2=w1252:i32[])  [unwired: 2 in]
              n859 = Index Array(array=w1260, index (row) #1=0 ("index (row)"), index (row) #2=1 ("index (row)")) -> (element #1=w1255:i32[], element #2=w1253:i32[])  [unwired: 2 in]
              n860 = Divide(x=w1255, y=w1254) -> (x/y=w1249:dbl[])
              n861 = Divide(x=w1253, y=w1252) -> (x/y=w1248:dbl[])
              n862 = Multiply(x=w1248, y=100.0 ("new element/subarray")) -> (x*y=w1243:dbl[])
              n863 = Multiply(x=100.0 ("new element/subarray"), y=w1249) -> (x*y=w1246:dbl[])
              n864 = Split 1D Array(array=w1246, index=22) -> (first subarray=→"comp_p1":dbl[], second subarray=→"comp_p1 2":dbl[])
              n865 = Split 1D Array(array=w1243, index=22) -> (first subarray=→"comp_p2":dbl[], second subarray=→"comp_p2 2":dbl[])
              n866 = case shown="\"2\"" "display\nselection" {
                tunnel: [w1399 w1400 w1401 w1402] -> w1267
                tunnel: w1266 -> [_ w1400 _ _]
                tunnel: w1169 -> [w1399 _ _ _]
                frame "1", Default {
                }
                frame "2" {
                }
                frame "3" {
                  n867 = local read "save1_data"() -> (w1401:dbl[][])
                }
                frame "4" {
                  n868 = local read "save2_data"() -> (w1402:dbl[][])
                }
              }
              n869 = Index Array(array=w1267, index (col) #1=37 ("disabled index (col)"), index (col) #2=38 ("index (col)")) -> (element #1=w1283:dbl[], element #2=w1280:dbl[])  [unwired: 2 in]
              n870 = for {
                N: 22 -> [_]
                tunnel: w1267 -> [w1449]
                tunnel: w1283 -> [w1448]
                tunnel: w1280 -> [w1447]
                tunnel: [w1445] -> w1281 mode=indexing
                tunnel: [w1444] -> w1282 mode=indexing
                i -> [w1442]
                n871 = Increment(x=w1442) -> (x+1=w1443:i32)
                n872 = Index Array(array=w1449, index (col)=w1443) -> (element=w1446:dbl[])  [unwired: 1 in]
                n873 = And(x=w1448, y=w1446) -> (x .and. y?=w1445:i32[])
                n874 = And(x=w1447, y=w1446) -> (x .and. y?=w1444:i32[])
              }
              n875 = Index Array(array=w1267, index (col) #1=23 ("disabled index (col)"), index (col) #2=25 ("index (col)"), index (col) #3=24 ("index (col)"), index (col) #4=26 ("index (col)")) -> (element #1=w1354:dbl[], element #2=w1359:dbl[], element #3=w1360:dbl[], element #4=w1358:dbl[])  [unwired: 4 in]
              n876 = Add Array Elements(numeric array=w1354) -> (sum=w1374:dbl)
              n877 = Add Array Elements(numeric array=w1360) -> (sum=w1373:dbl)
              n878 = local read "comp_p1 2"() -> (w1222:dbl[])
              n879 = local read "Compare"() -> (w1234:bool)
              n880 = local read "comp_p2 2"() -> (w1230:dbl[])
              n881 = Add Array Elements(numeric array=w1358) -> (sum=w1372:dbl)
              n882 = Add Array Elements(numeric array=w1359) -> (sum=w1375:dbl)
              n883 = local read "Compare"() -> (w1231:bool)
              n884 = Build Array(w1374, w1375) -> (w1233:dbl[])
              n885 = Build Array(w1373, w1372) -> (w1223:dbl[])
              n886 = Transpose 2D Array(2D array=w1281) -> (transposed array=w1292:i32[][])
              n887 = Transpose 2D Array(2D array=w1282) -> (transposed array=w1291:i32[][])
              n888 = Select(t=w1222, s=w1234, f=w1233) -> (s? t:f=w1232:dbl[])
              n889 = Select(t=w1230, s=w1231, f=w1223) -> (s? t:f=w1229:dbl[])
              n890 = for {
                N: 22 -> [_]
                tunnel: w1292 -> [w1441]
                tunnel: w1291 -> [w1440]
                tunnel: [w1437] -> w1182 mode=indexing
                tunnel: [w1436] -> w1168 mode=indexing
                i -> [w1439]
                n891 = Index Array(array=w1441, index (col)=w1439) -> (element=w1438:i32[])  [unwired: 1 in]
                n892 = Index Array(array=w1440, index (col)=w1439) -> (element=w1435:i32[])  [unwired: 1 in]
                n893 = Add Array Elements(numeric array=w1438) -> (sum=w1437:i32)
                n894 = Add Array Elements(numeric array=w1435) -> (sum=w1436:i32)
              }
              n895 = Number To Decimal String(number=w1232, width (-)=w1247) -> (decimal integer string=→"W1/E1":string[])
              n896 = Number To Decimal String(number=w1229, width (-)=w1247) -> (decimal integer string=→"W2/E2":string[])
              n897 = Split 1D Array(array=w1182, index=w1293) -> (first subarray=w1294:i32[], second subarray=w1170:i32[])
              n898 = Split 1D Array(array=w1168, index=w1298) -> (first subarray=w1297:i32[], second subarray=w1302:i32[])
              n899 = Insert Into Array(array=w1182, new element=w1222) -> (w1272:i32[])  [unwired: 1 in]
              n900 = Insert Into Array(array=w1168, new element=w1223) -> (w1271:i32[])  [unwired: 1 in]
              n901 = Add Array Elements(numeric array=w1297) -> (sum=w1296:i32)
              n902 = Add Array Elements(numeric array=w1294) -> (sum=w1295:i32)
              n903 = Build Array(w1272, w1271) -> (w1264:i32[][])
              n904 = Index Array(array=w1302, index #1=3 ("index"), index #2=4 ("index")) -> (element #1=w1290:i32, element #2=w1289:i32)
              n905 = Index Array(array=w1170, index #1=3 ("index"), index #2=4 ("index")) -> (element #1=w1299:i32, element #2=w1300:i32)
              n906 = for {
                N: w1293 -> [_]
                tunnel: w1294 -> [w1434] mode=indexing
                tunnel: w1295 -> [w1433]
                tunnel: [w1430] -> w1323 mode=indexing
                n907 = Divide(x=w1434, y=w1433) -> (x/y=w1432:dbl)
                n908 = Multiply(x=w1432, y=100.0) -> (x*y=w1430:dbl)
              }
              n909 = Add(x=w1290, y=w1289) -> (x+y=w1301:i32)
              n910 = for {
                N: w1298 -> [_]
                tunnel: w1297 -> [w1429] mode=indexing
                tunnel: w1296 -> [w1428]
                tunnel: [w1425] -> w1226 mode=indexing
                n911 = Divide(x=w1429, y=w1428) -> (x/y=w1427:dbl)
                n912 = Multiply(x=w1427, y=100.0) -> (x*y=w1425:dbl)
              }
              n913 = Add(x=w1299, y=w1300) -> (x+y=w1303:i32)
              n914 = case shown="\"1\"" "display\nselection" {
                tunnel: w1264 -> [_ w1398 _]
                frame "0", Default {
                }
                frame "1" {
                  "game" <- w1398
                }
                frame "2" {
                }
              }
              n915 = case shown="True" "save2 3" {
                tunnel: w1264 -> [_ w1405]
                tunnel: w1267 -> [_ w1403]
                frame False {
                }
                frame True {
                  n916 = local write "save2 3"(FALSE ("save2")) -> ()
                  "save2 2" <- w1405
                  "save2_data" <- w1403
                }
              }
              n917 = case shown="True" "save1 3" {
                tunnel: w1264 -> [_ w1408]
                tunnel: w1267 -> [_ w1406]
                frame False {
                }
                frame True {
                  n918 = local write "save1 3"(FALSE ("save1")) -> ()
                  "save1 2" <- w1408
                  "save1_data" <- w1406
                }
              }
              n919 = for {
                tunnel: w1302 -> [w1424] mode=indexing
                tunnel: w1301 -> [w1423]
                tunnel: [w1420] -> w1325 mode=indexing
                n920 = Divide(x=w1424, y=w1423) -> (x/y=w1422:dbl)
                n921 = Multiply(x=w1422, y=100.0) -> (x*y=w1420:dbl)
              }
              n922 = for {
                tunnel: w1170 -> [w1419] mode=indexing
                tunnel: w1303 -> [w1418]
                tunnel: [w1415] -> w1324 mode=indexing
                n923 = Divide(x=w1419, y=w1418) -> (x/y=w1417:dbl)
                n924 = Multiply(x=w1417, y=100.0) -> (x*y=w1415:dbl)
              }
              n925 = local read "comp_p2"() -> (w1238:dbl[])
              n926 = local read "Compare"() -> (w1237:bool)
              n927 = local read "comp_p1"() -> (w1239:dbl[])
              n928 = Insert Into Array(array=w1226, new element=w1325) -> (w1225:dbl[])  [unwired: 1 in]
              n929 = Insert Into Array(array=w1323, new element=w1324) -> (w1227:dbl[])  [unwired: 1 in]
              n930 = Select(t=w1238, s=w1237, f=w1225) -> (s? t:f=w1191:dbl[])
              n931 = Select(t=w1239, s="Compare", f=w1227) -> (s? t:f=w1186:dbl[])
              n932 = local read "Percentage"() -> (w1350:bool)
              n933 = local read "Percentage"() -> (w1351:bool)
              n934 = Split 1D Array(array=w1191, index=9) -> (second subarray=w1331:dbl[])  [unwired: 1 out]
              n935 = Number To Fractional String(number=w1191, precision (6)=i16 0) -> (F-format string=w1190:string[])  [unwired: 2 in]
              n936 = Split 1D Array(array=w1168, index=9) -> (second subarray=w1334:i32[])  [unwired: 1 out]
              n937 = Split 1D Array(array=w1186, index=9) -> (second subarray=w1330:dbl[])  [unwired: 1 out]
              n938 = Number To Fractional String(number=w1186, precision (6)=i16 0) -> (F-format string=w1183:string[])  [unwired: 2 in]
              n939 = Split 1D Array(array=w1182, index=9) -> (second subarray=w1328:i32[])  [unwired: 1 out]
              n940 = local read "Percentage"() -> (w1338:bool)
              n941 = Number To Fractional String(number=w1182, precision (6)=i16 0) -> (F-format string=w1184:string[])  [unwired: 2 in]
              n942 = Number To Decimal String(number=w1328, width (-)=i16 1 ("precision (6)")) -> (decimal integer string=w1337:string[])
              n943 = Number To Fractional String(number=w1168, precision (6)=i16 0) -> (F-format string=w1188:string[])  [unwired: 2 in]
              n944 = Number To Fractional String(number=w1330, precision (6)=i16 0) -> (F-format string=w1336:string[])  [unwired: 2 in]
              n945 = Number To Decimal String(number=w1334, width (-)=i16 1 ("precision (6)")) -> (decimal integer string=w1340:string[])
              n946 = Number To Fractional String(number=w1331, precision (6)=i16 0) -> (F-format string=w1339:string[])  [unwired: 2 in]
              n947 = Select(t=w1183, s=w1351, f=w1184) -> (s? t:f=w1172:string[])
              n948 = Select(t=w1336, s="Percentage", f=w1337) -> (s? t:f=w1208:string[])
              n949 = call "Search NaN_Inf (SubVI).vi"("in"=w1172) -> ("out"=w1171:string[])
              n950 = Select(t=w1339, s=w1338, f=w1340) -> (s? t:f=w1205:string[])
              n951 = Select(t=w1190, s=w1350, f=w1188) -> (s? t:f=w1192:string[])
              n952 = call "Search NaN_Inf (SubVI).vi"("in"=w1208) -> ("out"=w1207:string[])
              n953 = call "Search NaN_Inf (SubVI).vi"("in"=w1192) -> ("out"=w1195:string[])
              n954 = call "Search NaN_Inf (SubVI).vi"("in"=w1205) -> ("out"=w1206:string[])
              n955 = Insert Into Array(array=w1207, index=3, new element=w1345) -> (w1343:string[])
              n956 = Index Array(array=w1171, index #1=0 ("index"), index #2=1 ("index"), index #3=2 ("index"), index #4=3 ("index"), index #5=4 ("index"), index #6=5 ("index"), index #7=6 ("index"), index #8=7 ("index"), index #9=8 ("index")) -> (element #1=→"p1 1":string, element #2=→"p1 2":string, element #3=→"p1 3":string, element #4=→"p1 4":string, element #5=→"p1 5":string, element #6=→"p1 6":string, element #7=→"p1 7":string, element #8=→"p1 8":string, element #9=→"p1 9":string)
              n957 = Insert Into Array(array=w1206, index=3, new element=w1346) -> (w1348:string[])
              n958 = Insert Into Array(array=w1343, index=6, new element=w1345) -> (w1361:string[])
              n959 = Index Array(array=w1195, index #1=0 ("index"), index #2=1 ("index"), index #3=2 ("index"), index #4=3 ("index"), index #5=4 ("index"), index #6=5 ("index"), index #7=6 ("index"), index #8=7 ("index"), index #9=8 ("index")) -> (element #1=→"p2 17":string, element #2=→"p2 16":string, element #3=→"p2 12":string, element #4=→"p2 13":string, element #5=→"p2 15":string, element #6=→"p2 14":string, element #7=→"p2 10":string, element #8=→"p2 11":string, element #9=→"p2 9":string)
              n960 = Insert Into Array(array=w1348, index=6, new element=w1346) -> (w1369:string[])
              n961 = Split 1D Array(array=w1361, index=6) -> (first subarray=→"player1_2":string[], second subarray=w1364:string[])
              n962 = Split 1D Array(array=w1369, index=6) -> (first subarray=→"player2_2":string[], second subarray=w1367:string[])
              n963 = Delete From Array(array=w1364, index=0) -> (array with subset deleted=w1167:string[])  [unwired: 1 in, 1 out]
              "player12" <- w1167
              n964 = Delete From Array(array=w1367, index=0) -> (array with subset deleted=w1210:string[])  [unwired: 1 in, 1 out]
              "player2 2" <- w1210
              n965 = Fract/Exp String To Number(string=w1167) -> (number=w1204:dbl[])  [unwired: 3 in, 1 out]
              n966 = Fract/Exp String To Number(string=w1210) -> (number=w1203:dbl[])  [unwired: 3 in, 1 out]
              n967 = Array Max & Min(array=w1204) -> (max value=w1218:dbl)  [unwired: 3 out]
              n968 = Array Max & Min(array=w1203) -> (max value=w1217:dbl)  [unwired: 3 out]
              n969 = Interleave 1D Arrays(w1385, w1204) -> (w1221:dbl[])
              n970 = Insert Into Array(array=w1221, new element=0.0 ("new element/subarray")) -> (w1379:dbl[])  [unwired: 1 in]
              n971 = Max & Min(x=w1218, y=w1217) -> (max(x,y)=w1212:dbl)  [unwired: 1 out]
              n972 = Interleave 1D Arrays(w1385, w1203) -> (w1219:dbl[])
              n973 = Bundle(w1379, "array"=dbl[] [1.0, 2.0, 3.0, 4.0, 5.0, 6.0, 7.0, 8.0, 9.0, 10.0, 11.0, 12.0, 13.0, 14.0, 15.0, 16.0, 17.0]) -> (→"P1graph":cluster{dbl[], "array":dbl[]})  [unwired: 1 in]
              n974 = Equal?(x=w1212, y=inf) -> (x = y?=w1214:bool)
              n975 = Insert Into Array(array=w1219, new element=0.0 ("new element/subarray")) -> (w1380:dbl[])  [unwired: 1 in]
              n976 = Select(t=100.0, s=w1214, f=w1212) -> (s? t:f=w1211:dbl)
              n977 = Bundle(w1380, "array"=dbl[] [1.0, 2.0, 3.0, 4.0, 5.0, 6.0, 7.0, 8.0, 9.0, 10.0, 11.0, 12.0, 13.0, 14.0, 15.0, 16.0, 17.0]) -> (→"P2graph":cluster{dbl[], "array":dbl[]})  [unwired: 1 in]
              n978 = property on="P2graph" class="XYGraph (strict)"("XScale.Maximum"=w1211, "XScale.Minimum"=w1209) -> ()  [unwired: 2 in, 2 out]
              n979 = property on="P1graph" class="XYGraph (strict)"("XScale.Maximum"=w1211, "XScale.Minimum"=w1209) -> ()  [unwired: 2 in, 2 out]
              "Player 3" <- w1352
              "Player 1_2" <- w1352
              "Player 2_2" <- w1352
              "Player 4" <- w1352
              "W/E1" <- w1371
              "W/E2" <- w1371
            }
          }
          n980 = local read "refnum of data save file"() -> (w952:refnum<file>)
          n981 = local write "Code number display"(1 ("Code number")) -> ()
          n982 = Select(t=T1."Edit video" ("Main tab"), s="Extract data", f=T1."Display" ("Main tab")) -> (s? t:f=w959:T1)
          n983 = Select(t=T1."Examine coding" ("Main tab"), s="Examine code", f=w959) -> (s? t:f=w960:T1)
        }
        frame "Edit video" {
          w1450 = T4."Disabled and Grayed Out" ("Disabled")
          n984 = Build Array("TL", "TM", "TR", "CL", "CM", "CR", "BL", "BM", "BR", "FH 2", "BH 2", "OH 2", "ST", "CR 2", "smash", "defense", "drive", "lob", "drop", "chop", "clear", "net", "winner", "winner", "error", "error", "point 1", "point 2", "service1", "service2", "1 9", "2 9", "3 8", "4 8", "player1", "player2", "Button 6", "Button 7", "Button 8", "Button 9", "Button 10") -> (w1465:bool[])
          "Last Edit" <- w1465
          n985 = Delete From Array(array=w1463, length=2, index (col)=29 ("disabled index (col)")) -> (deleted portion=→"Score 2":i64[][], array with subset deleted=w1510:i64[][])  [unwired: 1 in]
          n986 = Index Array(array=w1510, index (col) #1=23 ("disabled index (col)"), index (col) #2=24 ("index (col)"), index (col) #3=25 ("index (col)"), index (col) #4=26 ("index (col)")) -> (element #1=w1520:i64[], element #2=w1519:i64[], element #3=w1518:i64[], element #4=w1517:i64[])  [unwired: 4 in]
          n987 = Or(x=w1518, y=w1517) -> (x .or. y?=w1511:i64[])
          n988 = Or(x=w1520, y=w1519) -> (x .or. y?=w1516:i64[])
          n989 = Replace Array Subset(array=w1510, new element #1=w1516, index (col) #1=23 ("disabled index (col)"), new element #2=w1516, index (col) #2=24 ("index (col)"), new element #3=w1511, index (col) #3=25 ("index (col)"), new element #4=w1511, index (col) #4=26 ("index (col)")) -> (w1509:i64[][])  [unwired: 4 in]
          n990 = property on="Code number display" class="DigNum (strict)"("DisabledEnum"=w1450) -> ()  [unwired: 2 in, 2 out]
          n991 = property on="Next" class="Bool (strict)"("DisabledEnum"=w1450) -> ()  [unwired: 2 in, 2 out]
          n992 = property on="Reset" class="Bool (strict)"("DisabledEnum"=w1450) -> ()  [unwired: 2 in, 2 out]
          n993 = property on="Update" class="Bool (strict)"("DisabledEnum"=w1450) -> ()  [unwired: 2 in, 2 out]
          n994 = property on="Previous" class="Bool (strict)"("DisabledEnum"=w1450) -> ()  [unwired: 2 in, 2 out]
          n995 = Delete From Array(array=w1509, length=1, index (col)=0 ("disabled index (col)")) -> (deleted portion=w1507:i64[][], array with subset deleted=w1508:i64[][])  [unwired: 1 in]
          "frame data" <- w1507
          "coded data" <- w1508
          n996 = Or Array Elements(Boolean array=w1465) -> (logical OR=w1506:bool)
          n997 = case shown="True" w1506 {
            tunnel: w1508 -> [_ w1578]
            tunnel: w1465 -> [_ w1574]
            tunnel: w1507 -> [w1548 w1573]
            tunnel: [w1551 w1562] -> w1500
            frame False {
              n998 = Delete From Array(array=w1548, length=1, index (col)=0 ("disabled index (col)")) -> (deleted portion=w1547:i64[][])  [unwired: 1 in, 1 out]
              n999 = Array Max & Min(array=w1547) -> (max value=w1549:i64, min value=w1550:i64)  [unwired: 2 out]
              n1000 = for {
                N: 300 -> [_]
                i -> [w1555]
                n1001 = Increment(x=w1555) -> (x+1=w1554:i32)
                n1002 = local write "task"(w1554) -> ()
                n1003 = Wait (ms)(milliseconds to wait=u32 1) -> ()  [unwired: 1 out]
              }
              n1004 = Build Array(w1550, w1549) -> (w1551:i64[])
            }
            frame True {
              n1005 = for {
                tunnel: w1574 -> [w1610] mode=indexing
                tunnel: w1578 -> [w1613]
                tunnel: [w1611] -> w1563 mode=indexing if=w1610
                i -> [w1612]
                n1006 = Index Array(array=w1613, index (col)=w1612) -> (element=w1611:i64[])  [unwired: 1 in]
              }
              n1007 = Transpose 2D Array(2D array=w1563) -> (transposed array=w1577:i64[][])
              n1008 = for {
                tunnel: w1573 -> [w1607] mode=indexing
                tunnel: w1577 -> [w1605] mode=indexing
                tunnel: [w1606] -> w1576 mode=indexing
                tunnel: [w1607] -> w1560 mode=indexing if=w1606
                n1009 = Array Max & Min(array=w1605) -> (min value=w1608:i64)  [unwired: 3 out]
                n1010 = Equal?(x=w1608, y=1) -> (x = y?=w1606:bool)
              }
              "edited\nevents" <- w1560
              n1011 = Index Array(array=w1560, index (col)=0 ("disabled index (col)")) -> (element=w1558:i64[])  [unwired: 1 in]
              n1012 = Array Size(array=w1558) -> (size(s)=w1557:i32)
              n1013 = Multiply(x="before", y=u32 25) -> (x*y=w1569:u32)
              n1014 = Multiply(x="after", y=u32 25) -> (x*y=w1570:u32)
              n1015 = Index Array(array=w1560, index (col)=0 ("disabled index (col)")) -> (element=w1572:i64[])  [unwired: 1 in]
              n1016 = property on="Code number display" class="DigNum (strict)"("Maximum"=w1557, "Minimum"=1.0 ("Data Entry Limits:Minimum")) -> ()  [unwired: 2 in, 2 out]
              n1017 = Or Array Elements(Boolean array=w1576) -> (logical OR=w1575:bool)
              n1018 = for {
                tunnel: w1569 -> [w1590]
                tunnel: w1570 -> [w1592]
                tunnel: w1572 -> [w1591] mode=indexing
                shift-right: [w1584] -> w1562
                shift-left: u32[] [] -> [w1586]
                n1019 = Array Max & Min(array=w1586) -> (max value=w1589:u32, max index (indices)=w1585:i32)  [unwired: 2 out]
                n1020 = Subtract(x=w1591, y=w1590) -> (x-y=w1588:i64)
                n1021 = Add(x=w1592, y=w1591) -> (x+y=w1587:i64)
                n1022 = Greater Or Equal?(x=w1589, y=w1588) -> (x >= y?=w1579:bool)
                n1023 = Build Array(w1588, w1587) -> (w1582:i64[])
                n1024 = Build Array(w1587) -> (w1583:i64[])
                n1025 = And(x="Combine", y=w1579) -> (x .and. y?=w1581:bool)
                n1026 = case shown="True" w1581 {
                  tunnel: w1586 -> [w1595 w1599]
                  tunnel: w1585 -> [_ w1598]
                  tunnel: w1583 -> [_ w1597]
                  tunnel: [w1594 w1596] -> w1584
                  tunnel: w1582 -> [w1593 _]
                  frame False {
                    n1027 = Insert Into Array(array=w1595, new element=w1593) -> (w1594:u32[])  [unwired: 1 in]
                  }
                  frame True {
                    n1028 = Replace Array Subset(array=w1599, new element=w1597, index=w1598) -> (w1596:u32[])
                  }
                }
              }
              n1029 = case shown="False" w1575 {
                frame False {
                  n1030 = One Button Dialog(message="This combination \nof events are \nnot available") -> ()  [unwired: 1 in, 1 out]
                }
                frame True {
                  n1031 = for {
                    N: 300 -> [_]
                    i -> [w1603]
                    n1032 = Increment(x=w1603) -> (x+1=w1602:i32)
                    n1033 = local write "task"(w1602) -> ()
                    n1034 = Wait (ms)(milliseconds to wait=u32 1) -> ()  [unwired: 1 out]
                  }
                }
              }
            }
          }
          "edited to play" <- w1500
          n1035 = local read "Btn 1"() -> (→"Btn 10":string)
          n1036 = local read "Btn 2"() -> (→"Btn 9":string)
          n1037 = local read "Btn 3"() -> (→"Btn 8":string)
          n1038 = local read "Btn 4"() -> (→"Btn 7":string)
          n1039 = local read "Btn 5"() -> (→"Btn 6":string)
          n1040 = local write "Extract data"(FALSE ("edit video")) -> ()
          n1041 = Array Size(array=w1500) -> (size(s)=w1505:i32)
          n1042 = Divide(x=w1505, y=2) -> (x/y=w1504:dbl)
          n1043 = for {
            N: w1504 -> [_]
            shift-right: [w1536] -> _
            shift-left: w1500 -> [w1538]
            shift-right: [w1531] -> w1501
            shift-left: i64[] [] ("edited\nto play 3") -> [w1532]
            n1044 = Split 1D Array(array=w1538, index=2) -> (first subarray=w1537:i64[], second subarray=w1536:i64[])
            n1045 = Index Array(array=w1537, index #1=1 ("index"), index #2=0 ("index")) -> (element #1=w1542:i64, element #2=w1535:i64)
            n1046 = Subtract(x=w1542, y=w1535) -> (x-y=w1534:i64)
            n1047 = Increment(x=w1534) -> (x+1=w1533:i64)
            n1048 = for {
              N: w1533 -> [_]
              tunnel: w1535 -> [w1545]
              tunnel: [w1543] -> w1530 mode=indexing
              i -> [w1544]
              n1049 = Add(x=w1545, y=w1544) -> (x+y=w1543:i64)
            }
            n1050 = Insert Into Array(array=w1532, new element=w1530) -> (w1531:i64[])  [unwired: 1 in]
          }
          "frames edited" <- w1501
          "frames 2 play" <- w1501
          n1051 = local read "refnum of data save file"() -> (w1461:refnum<file>)
        }
        frame "Examine coding" {
          w1614 = T4."Enabled" ("Disabled")
          n1052 = property on="Code number display" class="DigNum (strict)"("DisabledEnum"=w1614) -> ()  [unwired: 2 in, 2 out]
          n1053 = property on="Next" class="Bool (strict)"("DisabledEnum"=w1614) -> ()  [unwired: 2 in, 2 out]
          n1054 = property on="Reset" class="Bool (strict)"("DisabledEnum"=w1614) -> ()  [unwired: 2 in, 2 out]
          n1055 = property on="Update" class="Bool (strict)"("DisabledEnum"=w1614) -> ()  [unwired: 2 in, 2 out]
          n1056 = property on="Previous" class="Bool (strict)"("DisabledEnum"=w1614) -> ()  [unwired: 2 in, 2 out]
          n1057 = local read "edited\nevents"() -> (w1627:i64[][])
          n1058 = Decrement(x="Code number display") -> (x-1=w1615:i32)
          n1059 = flat-sequence {
            tunnel: "Code number display" -> [w1683]
            frame #0 {
              n1060 = local read "edited to play"() -> (w1682:i64[])
              n1061 = for {
                N: w1683 -> [_]
                shift-right: [w1688] -> _
                shift-left: w1682 -> [w1689]
                tunnel: [w1687] -> w1675
                n1062 = Split 1D Array(array=w1689, index=2) -> (first subarray=w1687:i64[], second subarray=w1688:i64[])
              }
              n1063 = Index Array(array=w1675, index #1=1 ("index"), index #2=0 ("index")) -> (element #1=w1681:i64, element #2=w1678:i64)
              n1064 = Subtract(x=w1681, y=w1678) -> (x-y=w1677:i64)
              n1065 = Increment(x=w1677) -> (x+1=w1676:i64)
              n1066 = for {
                N: w1676 -> [_]
                tunnel: w1678 -> [w1686]
                tunnel: [w1684] -> w1674 mode=indexing
                i -> [w1685]
                n1067 = Add(x=w1686, y=w1685) -> (x+y=w1684:i64)
              }
              n1068 = local write "Progress..."(u32 0 ("Progress...")) -> ()
              n1069 = local write "frames 2 play"(w1674) -> ()
            }
            frame #1 {
              w1691 = TRUE ("Play")
              w1692 = FALSE ("Next")
              n1070 = local write "Next"(w1692) -> ()
              n1071 = local write "Previous"(w1692) -> ()
              n1072 = local write "Reset"(w1692) -> ()
              n1073 = local write "stop"(w1692) -> ()
              n1074 = local write "Pause"(w1692) -> ()
              n1075 = local write "Load video"(w1691) -> ()
              n1076 = local write "Play"(w1691) -> ()
            }
          }
          n1077 = Index Array(array=w1627, index (row)=w1615, index (col)=0) -> (element=w1626:i64)
          n1078 = Index Array(array=w1624, index (col)=0 ("disabled index (col)")) -> (element=w1670:i64[])  [unwired: 1 in]
          n1079 = Search 1D Array(1D array=w1670, element=w1626) -> (index of element=w1669:i32)  [unwired: 1 in]
          n1080 = Index Array(array=w1624, index (row)=w1669) -> (element=w1668:i64[])  [unwired: 1 in]
          n1081 = Delete From Array(array=w1668, index=0) -> (array with subset deleted=w1667:i64[])  [unwired: 1 in, 1 out]
          n1082 = for {
            tunnel: w1667 -> [w1697] mode=indexing
            tunnel: [w1693] -> w1666 mode=indexing
            n1083 = Equal To 0?(x=w1697) -> (x = 0?=w1696:bool)
            n1084 = Select(t=FALSE ("x = 0?"), s=w1696, f=TRUE) -> (s? t:f=w1693:bool)
          }
          n1085 = Index Array(array=w1666) -> (element #1=w1665:bool, element #2=w1664:bool, element #3=w1663:bool, element #4=w1662:bool, element #5=w1661:bool, element #6=w1660:bool, element #7=w1659:bool, element #8=w1658:bool, element #9=w1657:bool, element #10=w1656:bool, element #11=w1655:bool, element #12=w1654:bool, element #13=w1653:bool, element #14=w1652:bool, element #15=w1651:bool, element #16=w1650:bool, element #17=w1649:bool, element #18=w1648:bool, element #19=w1647:bool, element #20=w1646:bool, element #21=w1645:bool, element #22=w1644:bool, element #23=w1643:bool, element #24=w1642:bool, element #25=w1641:bool, element #26=w1640:bool, element #27=w1637:bool, element #28=w1636:bool, element #31=w1635:bool, element #32=w1634:bool, element #33=w1633:bool, element #34=w1632:bool, element #35=w1631:bool, element #36=w1630:bool, element #37=w1629:bool, element #38=w1628:bool, element #39=w1621:bool, element #40=w1620:bool, element #41=w1619:bool, element #42=w1618:bool, element #43=w1617:bool)  [unwired: 43 in, 2 out]
          n1086 = Or(x=w1643, y=w1642) -> (x .or. y?=w1639:bool)
          n1087 = Or(x=w1641, y=w1640) -> (x .or. y?=w1638:bool)
          n1088 = local write "TL"(w1665) -> ()
          n1089 = local write "TM"(w1664) -> ()
          n1090 = local write "TR"(w1663) -> ()
          n1091 = local write "CL"(w1662) -> ()
          n1092 = local write "CM"(w1661) -> ()
          n1093 = local write "CR"(w1660) -> ()
          n1094 = local write "BL"(w1659) -> ()
          n1095 = local write "BM"(w1658) -> ()
          n1096 = local write "BR"(w1657) -> ()
          n1097 = local write "FH 2"(w1656) -> ()
          n1098 = local write "BH 2"(w1655) -> ()
          n1099 = local write "OH 2"(w1654) -> ()
          n1100 = local write "ST"(w1653) -> ()
          n1101 = local write "CR 2"(w1652) -> ()
          n1102 = local write "smash"(w1651) -> ()
          n1103 = local write "defense"(w1650) -> ()
          n1104 = local write "drive"(w1649) -> ()
          n1105 = local write "drop"(w1647) -> ()
          n1106 = local write "chop"(w1646) -> ()
          n1107 = local write "clear"(w1645) -> ()
          n1108 = local write "net"(w1644) -> ()
          n1109 = local write "winner"(w1639) -> ()
          n1110 = local write "error"(w1638) -> ()
          n1111 = local write "point 1"(w1637) -> ()
          n1112 = local write "point 2"(w1636) -> ()
          n1113 = local write "service1"(w1635) -> ()
          n1114 = local write "service2"(w1634) -> ()
          n1115 = local write "1 9"(w1633) -> ()
          n1116 = local write "2 9"(w1632) -> ()
          n1117 = local write "3 8"(w1631) -> ()
          n1118 = local write "4 8"(w1630) -> ()
          n1119 = local write "player1"(w1629) -> ()
          n1120 = local write "player2"(w1628) -> ()
          n1121 = local write "Button 6"(w1621) -> ()
          n1122 = local write "Button 7"(w1620) -> ()
          n1123 = local write "Button 8"(w1619) -> ()
          n1124 = local write "Button 9"(w1618) -> ()
          n1125 = local write "Button 10"(w1617) -> ()
          n1126 = local write "lob"(w1648) -> ()
          n1127 = local read "refnum of data save file"() -> (w1622:refnum<file>)
        }
        frame "Edit coding" {
          n1128 = local read "Examine code"() -> (w1699:bool)
          n1129 = case shown="True" w1699 {
            tunnel: [T1."Edit video" ("Main tab") w1750] -> w1701
            frame False {
              n1130 = local read "Last Edit"() -> (w1716:bool[])
              n1131 = Index Array(array=w1716) -> (element #1=w1746:bool, element #2=w1745:bool, element #3=w1744:bool, element #4=w1743:bool, element #5=w1742:bool, element #6=w1741:bool, element #7=w1740:bool, element #8=w1739:bool, element #9=w1738:bool, element #10=w1737:bool, element #11=w1736:bool, element #12=w1735:bool, element #13=w1734:bool, element #14=w1733:bool, element #15=w1732:bool, element #16=w1731:bool, element #17=w1730:bool, element #18=w1729:bool, element #19=w1728:bool, element #20=w1727:bool, element #21=w1726:bool, element #22=w1725:bool, element #23=w1724:bool, element #24=w1723:bool, element #25=w1722:bool, element #26=w1721:bool, element #27=w1718:bool, element #28=w1717:bool, element #29=w1714:bool, element #30=w1713:bool, element #31=w1712:bool, element #32=w1711:bool, element #33=w1710:bool, element #34=w1709:bool, element #35=w1708:bool, element #36=w1707:bool, element #37=w1706:bool, element #38=w1705:bool, element #39=w1704:bool, element #40=w1703:bool, element #41=w1702:bool)  [unwired: 41 in]
              n1132 = Or(x=w1724, y=w1723) -> (x .or. y?=w1720:bool)
              n1133 = Or(x=w1722, y=w1721) -> (x .or. y?=w1719:bool)
              n1134 = local write "TL"(w1746) -> ()
              n1135 = local write "TM"(w1745) -> ()
              n1136 = local write "TR"(w1744) -> ()
              n1137 = local write "CL"(w1743) -> ()
              n1138 = local write "CM"(w1742) -> ()
              n1139 = local write "CR"(w1741) -> ()
              n1140 = local write "BL"(w1740) -> ()
              n1141 = local write "BM"(w1739) -> ()
              n1142 = local write "BR"(w1738) -> ()
              n1143 = local write "FH 2"(w1737) -> ()
              n1144 = local write "BH 2"(w1736) -> ()
              n1145 = local write "OH 2"(w1735) -> ()
              n1146 = local write "ST"(w1734) -> ()
              n1147 = local write "CR 2"(w1733) -> ()
              n1148 = local write "smash"(w1732) -> ()
              n1149 = local write "defense"(w1731) -> ()
              n1150 = local write "drive"(w1730) -> ()
              n1151 = local write "drop"(w1728) -> ()
              n1152 = local write "chop"(w1727) -> ()
              n1153 = local write "clear"(w1726) -> ()
              n1154 = local write "net"(w1725) -> ()
              n1155 = local write "winner"(w1720) -> ()
              n1156 = local write "error"(w1719) -> ()
              n1157 = local write "point 1"(w1718) -> ()
              n1158 = local write "point 2"(w1717) -> ()
              n1159 = local write "service1"(w1714) -> ()
              n1160 = local write "service2"(w1713) -> ()
              n1161 = local write "1 9"(w1712) -> ()
              n1162 = local write "2 9"(w1711) -> ()
              n1163 = local write "3 8"(w1710) -> ()
              n1164 = local write "4 8"(w1709) -> ()
              n1165 = local write "player1"(w1708) -> ()
              n1166 = local write "player2"(w1707) -> ()
              n1167 = local write "Button 6"(w1706) -> ()
              n1168 = local write "Button 7"(w1705) -> ()
              n1169 = local write "Button 8"(w1704) -> ()
              n1170 = local write "Button 9"(w1703) -> ()
              n1171 = local write "Button 10"(w1702) -> ()
              n1172 = local write "lob"(w1729) -> ()
              n1173 = local write "Upload edited video"(TRUE ("Upload edited video")) -> ()
            }
            frame True {
              n1174 = event shown="[0] Timeout" {
                selector: _ -> [_ _]
                dyn-events: _ -> [_ _]
                timeout: 25 -> [_ _]
                tunnel: [FALSE TRUE] -> w1748
                event Timeout {
                  n1175 = event-data() -> ()  [unwired: 1 in, 3 out]
                }
                event "Code number display": Value Change {
                  n1176 = event-data() -> ()  [unwired: 1 in, 3 out]
                }
              }
              n1177 = case shown="True" "Next" {
                frame False {
                }
                frame True {
                  n1178 = local read "edited\nevents"() -> (w1767:i64[][])
                  n1179 = local read "Code number display"() -> (w1763:i32)
                  n1180 = Index Array(array=w1767, index (col)=0 ("disabled index (col)")) -> (element=w1769:i64[])  [unwired: 1 in]
                  n1181 = Array Size(array=w1769) -> (size(s)=w1762:i32)
                  n1182 = Increment(x=w1763) -> (x+1=w1765:i32)
                  n1183 = Less Or Equal?(x=w1765, y=w1762) -> (x <= y?=w1766:bool)
                  n1184 = Select(t=w1765, s=w1766, f=w1762) -> (s? t:f=w1764:i32)
                  n1185 = local write "Code number display"(w1764) -> ()
                }
              }
              n1186 = case shown="True" "Previous" {
                frame False {
                }
                frame True {
                  n1187 = local read "Code number display"() -> (w1770:i32)
                  n1188 = Decrement(x=w1770) -> (x-1=w1773:i32)
                  n1189 = Greater Than 0?(x=w1773) -> (x > 0?=w1774:bool)
                  n1190 = Select(t=w1773, s=w1774, f=1) -> (s? t:f=w1771:i32)
                  n1191 = local write "Code number display"(w1771) -> ()
                }
              }
              n1192 = Compound Arithmetic op=OR(w1748, "Reset", "Previous", "Next") -> (w1756:bool)
              n1193 = Select(t=T1."Examine coding" ("Main tab"), s=w1756, f=T1."Edit coding" ("Main tab")) -> (s? t:f=w1751:T1)
              n1194 = Select(t=T1."Update coding" ("Main tab"), s="Update", f=w1751) -> (s? t:f=w1750:T1)
            }
          }
          n1195 = local read "refnum of data save file"() -> (w1698:refnum<file>)
        }
        frame "Update coding" {
          w1787 = "\r"
          n1196 = flat-sequence {
            tunnel: w1792 -> [w1804]
            tunnel: [w1801] -> w1791
            tunnel: w1791 -> [w1869]
            tunnel: [w1869] -> w1777
            frame #0 {
              w1818 = FALSE ("element")
              n1197 = local read "player1"() -> (w1817:bool)
              n1198 = local read "player2"() -> (w1805:bool)
              n1199 = local read "point 1"() -> (w1854:bool)
              n1200 = local read "point 2"() -> (w1853:bool)
              n1201 = local read "winner"() -> (w1816:bool)
              n1202 = local read "error"() -> (w1855:bool)
              n1203 = local read "service1"() -> (w1824:bool)
              n1204 = local read "service2"() -> (w1823:bool)
              n1205 = local read "defense"() -> (w1837:bool)
              n1206 = local read "smash"() -> (w1838:bool)
              n1207 = local read "OH 2"() -> (w1841:bool)
              n1208 = local read "chop"() -> (w1833:bool)
              n1209 = local read "drive"() -> (w1836:bool)
              n1210 = local read "BH 2"() -> (w1842:bool)
              n1211 = local read "drop"() -> (w1834:bool)
              n1212 = local read "clear"() -> (w1832:bool)
              n1213 = local read "FH 2"() -> (w1843:bool)
              n1214 = local read "CR 2"() -> (w1839:bool)
              n1215 = local read "CM"() -> (w1848:bool)
              n1216 = local read "TM"() -> (w1851:bool)
              n1217 = local read "BM"() -> (w1845:bool)
              n1218 = local read "lob"() -> (w1835:bool)
              n1219 = local read "net"() -> (w1831:bool)
              n1220 = local read "CR"() -> (w1847:bool)
              n1221 = local read "1 9"() -> (w1822:bool)
              n1222 = local read "2 9"() -> (w1821:bool)
              n1223 = local read "3 8"() -> (w1820:bool)
              n1224 = local read "4 8"() -> (w1819:bool)
              n1225 = local read "TR"() -> (w1850:bool)
              n1226 = local read "CL"() -> (w1849:bool)
              n1227 = local read "BR"() -> (w1844:bool)
              n1228 = local read "TL"() -> (w1852:bool)
              n1229 = local read "BL"() -> (w1846:bool)
              n1230 = local read "ST"() -> (w1840:bool)
              n1231 = And(x=w1817, y=w1816) -> (x .and. y?=w1830:bool)
              n1232 = And(x=w1805, y=w1816) -> (x .and. y?=w1829:bool)
              n1233 = And(x=w1817, y=w1855) -> (x .and. y?=w1828:bool)
              n1234 = And(x=w1805, y=w1855) -> (x .and. y?=w1827:bool)
              n1235 = Compound Arithmetic op=OR(w1827, w1830, w1854) -> (w1826:bool)
              n1236 = Compound Arithmetic op=OR(w1829, w1828, w1853) -> (w1825:bool)
              n1237 = local read "Button 10"() -> (w1796:bool)
              n1238 = local read "Button 6"() -> (w1800:bool)
              n1239 = local read "Button 7"() -> (w1799:bool)
              n1240 = local read "Button 8"() -> (w1798:bool)
              n1241 = local read "Button 9"() -> (w1797:bool)
              n1242 = Build Array(w1852, w1851, w1850, w1849, w1848, w1847, w1846, w1845, w1844, w1843, w1842, w1841, w1840, w1839, w1838, w1837, w1836, w1835, w1834, w1833, w1832, w1831, w1830, w1829, w1828, w1827, w1826, w1825, w1818, w1818, w1824, w1823, w1822, w1821, w1820, w1819, w1817, w1805, w1800, w1799, w1798, w1797, w1796) -> (w1815:bool[])
              n1243 = Boolean To (0,1)(Boolean=w1815) -> (0, 1=w1807:i16[])
              n1244 = local read "Code number display"() -> (w1795:i32)
              n1245 = local read "edited\nevents"() -> (w1808:i64[][])
              n1246 = Decrement(x=w1795) -> (x-1=w1794:i32)
              n1247 = Index Array(array=w1804, index (col)=0 ("disabled index (col)")) -> (element=w1812:i64[])  [unwired: 1 in]
              n1248 = Index Array(array=w1808, index (row)=w1794, index (col)=0) -> (element=w1810:i64)
              n1249 = Search 1D Array(1D array=w1812, element=w1810) -> (index of element=w1802:i32)  [unwired: 1 in]
              n1250 = Index Array(array=w1804, index (row)=w1802) -> (element=w1811:i64[])  [unwired: 1 in]
              n1251 = Delete From Array(array=w1811, index=0) -> (deleted portion=w1806:i64)  [unwired: 1 in, 1 out]
              n1252 = Build Array (concatenate)(w1806, w1807) -> (w1803:i64[])
              n1253 = Replace Array Subset(array=w1804, new element=w1803, index (row)=w1802) -> (w1801:i64[][])  [unwired: 1 in]
            }
            frame #1 {
              n1254 = local read "Last Edit"() -> (w1900:bool[])
              n1255 = Index Array(array=w1900) -> (element #1=w1870:bool, element #2=w1871:bool, element #3=w1872:bool, element #4=w1873:bool, element #5=w1874:bool, element #6=w1875:bool, element #7=w1876:bool, element #8=w1877:bool, element #9=w1878:bool, element #10=w1879:bool, element #11=w1880:bool, element #12=w1881:bool, element #13=w1882:bool, element #14=w1883:bool, element #15=w1884:bool, element #16=w1885:bool, element #17=w1886:bool, element #18=w1887:bool, element #19=w1888:bool, element #20=w1889:bool, element #21=w1890:bool, element #22=w1891:bool, element #23=w1892:bool, element #24=w1893:bool, element #25=w1894:bool, element #26=w1895:bool, element #27=w1898:bool, element #28=w1899:bool, element #29=w1868:bool, element #30=w1867:bool, element #31=w1866:bool, element #32=w1865:bool, element #33=w1864:bool, element #34=w1863:bool, element #35=w1862:bool, element #36=w1861:bool, element #37=w1860:bool, element #38=w1859:bool, element #39=w1858:bool, element #40=w1857:bool, element #41=w1856:bool)  [unwired: 41 in]
              n1256 = Or(x=w1892, y=w1893) -> (x .or. y?=w1896:bool)
              n1257 = Or(x=w1894, y=w1895) -> (x .or. y?=w1897:bool)
              n1258 = local write "TL"(w1870) -> ()
              n1259 = local write "TM"(w1871) -> ()
              n1260 = local write "TR"(w1872) -> ()
              n1261 = local write "CL"(w1873) -> ()
              n1262 = local write "CM"(w1874) -> ()
              n1263 = local write "CR"(w1875) -> ()
              n1264 = local write "BL"(w1876) -> ()
              n1265 = local write "BM"(w1877) -> ()
              n1266 = local write "BR"(w1878) -> ()
              n1267 = local write "FH 2"(w1879) -> ()
              n1268 = local write "BH 2"(w1880) -> ()
              n1269 = local write "OH 2"(w1881) -> ()
              n1270 = local write "ST"(w1882) -> ()
              n1271 = local write "CR 2"(w1883) -> ()
              n1272 = local write "smash"(w1884) -> ()
              n1273 = local write "defense"(w1885) -> ()
              n1274 = local write "drive"(w1886) -> ()
              n1275 = local write "drop"(w1888) -> ()
              n1276 = local write "chop"(w1889) -> ()
              n1277 = local write "clear"(w1890) -> ()
              n1278 = local write "net"(w1891) -> ()
              n1279 = local write "winner"(w1896) -> ()
              n1280 = local write "error"(w1897) -> ()
              n1281 = local write "point 1"(w1898) -> ()
              n1282 = local write "point 2"(w1899) -> ()
              n1283 = local write "service1"(w1868) -> ()
              n1284 = local write "service2"(w1867) -> ()
              n1285 = local write "1 9"(w1866) -> ()
              n1286 = local write "2 9"(w1865) -> ()
              n1287 = local write "3 8"(w1864) -> ()
              n1288 = local write "4 8"(w1863) -> ()
              n1289 = local write "player1"(w1862) -> ()
              n1290 = local write "player2"(w1861) -> ()
              n1291 = local write "lob"(w1887) -> ()
              n1292 = local write "Button 6"(w1860) -> ()
              n1293 = local write "Button 7"(w1859) -> ()
              n1294 = local write "Button 8"(w1858) -> ()
              n1295 = local write "Button 9"(w1857) -> ()
              n1296 = local write "Button 10"(w1856) -> ()
            }
          }
          n1297 = call "EVENTS(SubVI).vi"() -> ("Events"=w1785:string)  [unwired: 1 in]
          n1298 = local read "Video file"() -> (w1783:path)
          n1299 = local read "Data file"() -> (w1776:path)
          n1300 = call <vilib>:"Get File Extension.vi"("file"=w1783) -> ("filename without extension"=w1786:string)  [unwired: 7 in, 3 out]
          n1301 = Array To Spreadsheet String(delimiter (Tab)="\t" ("delimiter (\\t)"), array=w1777, 3:"%.3f" ("format (%.3f)")) -> (spreadsheet string=w1789:string)
          n1302 = Open/Create/Replace File(file path (use dialog)=w1776, operation (0:open)=T3."replace") -> (refnum out=w1779:refnum<file>, error out=w1778:errorcluster)  [unwired: 4 in, 1 out]
          n1303 = Concatenate Strings("avi file" ("string"), w1787, w1786, w1787, w1787, w1785, w1789) -> (w1788:string)
          n1304 = Write to Text File(file (use dialog)=w1779, text=w1788, error in=w1778) -> (refnum out=w1775:refnum<file>)  [unwired: 1 in, 2 out]
          n1305 = local write "Update"(FALSE ("Update")) -> ()
        }
      }
      "refnum of data save file" <- w374
      n1306 = Equal?(x="Main tab", y=enum32{"Coding", "Display"}."Coding" ("Tab Control 3")) -> (x = y?=w384:bool)
      n1307 = Not Equal?(x=w373, y=w379) -> (x != y?=w383:bool)
      n1308 = Select(t=w379, s=w384, f=w381) -> (s? t:f=w372:T1)
      n1309 = And(x=w383, y=w384) -> (x .and. y?=w382:bool)
      n1310 = Equal?(x=w373, y=w379) -> (x = y?=w378:bool)
      n1311 = Equal?(x=w372, y=w381) -> (x = y?=w380:bool)
      n1312 = And(x=w380, y=w378) -> (x .and. y?=w377:bool)
      n1313 = case shown="True" w382 {
        tunnel: w376 -> [_ w393]
        frame False {
        }
        frame True {
          # "Moving back to coding tab"
          n1314 = flat-sequence {
            tunnel: w393 -> [w397]
            frame #0 {
              n1315 = local read "ful video frames"() -> (w398:i64[])
              n1316 = Index Array(array=w397, index (col)=0 ("disabled index (col)")) -> (element=w395:i64[])  [unwired: 1 in]
              n1317 = Array Max & Min(array=w395) -> (max value=w394:i64)  [unwired: 3 out]
              n1318 = local write "frames 2 play"(w398) -> ()
              n1319 = local write "Progress..."(w394) -> ()
            }
            frame #1 {
              w399 = FALSE ("Next")
              w400 = TRUE ("Play")
              n1320 = local write "stop"(w400) -> ()
              n1321 = local write "Load video"(w400) -> ()
              n1322 = local write "Pause"(w399) -> ()
              n1323 = local write "Update"(w399) -> ()
              n1324 = local write "Next"(w399) -> ()
              n1325 = local write "Previous"(w399) -> ()
              n1326 = local write "Reset"(w399) -> ()
              n1327 = local write "Extract data"(w399) -> ()
              n1328 = local write "Upload edited video"(w399) -> ()
              n1329 = local write "Examine code"(w399) -> ()
            }
          }
        }
      }
      n1330 = case shown="True" w377 {
        frame False {
        }
        frame True {
          n1331 = local write "Progress..."(u32 0 ("Progress...")) -> ()
          n1332 = local write "Pause"(FALSE ("Pause")) -> ()
          n1333 = local write "stop"(TRUE ("stop")) -> ()
        }
      }
      n1334 = local read "START"() -> (w375:bool)
      n1335 = Wait (ms)(milliseconds to wait=u32 200) -> ()  [unwired: 1 out]
      "Main tab 2" <- w373
    }
    n1336 = while {
      tunnel: w10 -> [w223]
      tunnel: w1 -> [_]
      tunnel: [w218] -> w5
      stop <- w218 continue-if-true
      # "This loop is for writing\nvideo to disk"
      n1337 = local read "Video files to write"() -> (w222:string[])
      n1338 = local read "frames to write"() -> (w220:i64[][])
      n1339 = case shown="True" "Write file" {
        tunnel: [FALSE FALSE] -> w225
        tunnel: w223 -> [_ w243]
        tunnel: w222 -> [_ w242]
        tunnel: "Video to write" -> [_ w241]
        tunnel: w220 -> [_ w240]
        tunnel: [u32 0 ("milliseconds to wait") u32 0 ("milliseconds to wait")] -> w219
        frame False {
          w227 = T4."Enabled" ("Disabled")
          n1340 = local read "Video files to write"() -> (w231:string[])
          n1341 = property on="Add to lib" class="Bool (strict)"("DisabledEnum"=w227) -> ()  [unwired: 2 in, 2 out]
          n1342 = property on="File name" class="Str"("DisabledEnum"=w227) -> ()  [unwired: 2 in, 2 out]
          n1343 = property on="Video to write" class="Path"("DisabledEnum"=w227) -> ()  [unwired: 2 in, 2 out]
          n1344 = property on="START" class="Bool (strict)"("DisabledEnum"=w227) -> ()  [unwired: 2 in, 2 out]
          n1345 = Empty Array?(array=w231) -> (empty?=w230:bool)
          n1346 = Select(t=T4."Disabled and Grayed Out" ("Disabled"), s=w230, f=w227) -> (s? t:f=w228:T4)
          n1347 = property on="Write file" class="Bool (strict)"("DisabledEnum"=w228) -> ()  [unwired: 2 in, 2 out]
          n1348 = local write "Abort"(FALSE ("Abort")) -> ()
        }
        frame True {
          w235 = T4."Disabled and Grayed Out" ("Disabled")
          n1349 = for {
            tunnel: w240 -> [w282] mode=indexing
            tunnel: w242 -> [w273] mode=indexing
            tunnel: w241 -> [w272]
            tunnel: w243 -> [w260]
            tunnel: [w254] -> w238
            tunnel: [w253] -> w237
            tunnel: [w251] -> w236
            i -> [w255]
            stop <- w252 stop-if-true
            w269 = T5 4 items=["Grayscale (U8)", "Grayscale (I16)", "Grayscale (SGL)", "Complex (CSG)", "RGB (U32)", "HSL (U32)", "RGB (U64)"] ("Image Type")
            n1350 = Path To String(path=w272) -> (string=w274:string)
            n1351 = for {
              tunnel: w282 -> [w320] mode=indexing
              tunnel: [w320] -> w259 mode=indexing if=w319
              n1352 = Not Equal To 0?(x=w320) -> (x != 0?=w319:bool)
            }
            n1353 = Concatenate Strings(w274, "\\" ("string"), w273) -> (w277:string)
            n1354 = Array Size(array=w259) -> (size(s)=w258:i32)
            n1355 = Decrement(x=w255) -> (x-1=w256:i32)
            n1356 = Not Equal To 0?(x=w255) -> (x != 0?=w257:bool)
            n1357 = call <vilib>:"Search and Replace Pattern.vi"("string"=w277, "regular expression (\"\")"=".avi" ("regular expression (\"\")")) -> ("result string"=w281:string)  [unwired: 3 in, 1 out]
            n1358 = case shown="True" w257 {
              tunnel: w256 -> [_ w292]
              frame False {
              }
              frame True {
                n1359 = local read "Video files to write"() -> (w296:string[])
                n1360 = local read "frames to write"() -> (w293:i64[][])
                n1361 = Delete From Array(array=w296, index=w292) -> (array with subset deleted=w295:string[])  [unwired: 1 in, 1 out]
                n1362 = Delete From Array(array=w293, index (row)=w292) -> (array with subset deleted=w294:i64[][])  [unwired: 2 in, 1 out]
                n1363 = local write "frames to write"(w294) -> ()
                n1364 = local write "Video files to write"(w295) -> ()
              }
            }
            n1365 = property on="Writing" class="Slide (strict)"("Scale.Maximum"=w258) -> ()  [unwired: 2 in, 2 out]
            n1366 = Concatenate Strings(w281, ".avi" ("string")) -> (w279:string)
            n1367 = String To Path(string=w279) -> (path=w280:path)
            n1368 = while {
              shift-right: [w300] -> _
              shift-left: w280 -> [w299]
              tunnel: w281 -> [w304]
              tunnel: [w299] -> w250
              i -> [w298]
              stop <- w306 continue-if-true
              n1369 = Increment(x=w298) -> (x+1=w297:i32)
              n1370 = call <vilib>:"Check if File or Folder Exists.vi"("path"=w299) -> ("file or folder exists?"=w306:bool)  [unwired: 8 in, 2 out]
              n1371 = Number To Decimal String(number=w297) -> (decimal integer string=w303:string)  [unwired: 1 in]
              n1372 = Concatenate Strings(w304, " (file path clash) - " ("string"), w303, ".avi" ("string")) -> (w301:string)
              n1373 = String To Path(string=w301) -> (path=w300:path)
            }
            n1374 = Select(t="Microsoft Video 1" ("Codec Name"), s="Video compress", f="" ("Codec Name")) -> (s? t:f=w246:string)
            n1375 = local read "framesPerSecond"() -> (w263:u32)
            n1376 = call "IMAQ AVI Create"("Compression Filter"=w246, "Frames Per Second"=w263, "AVI Path"=w250) -> ("error out"=w270:errorcluster, "Avi Refnum"=w264:T6)  [unwired: 7 in]
            n1377 = call "IMAQ Create"("Image Name"="write", "Image Type"=w269, "error in (no error)"=w270) -> ("New Image"=w268:T2, "error out"=w267:errorcluster)  [unwired: 2 in]
            n1378 = for {
              tunnel: w259 -> [w317] mode=indexing
              tunnel: w268 -> [w311]
              tunnel: w267 -> [w316]
              tunnel: [w314] -> w266
              tunnel: [w313] -> w265
              tunnel: w264 -> [w312]
              tunnel: [w311] -> w261
              tunnel: w260 -> [w310]
              tunnel: ["Abort"] -> w252
              i -> [w309]
              stop <- "Abort" stop-if-true
              n1379 = Increment(x=w309) -> (x+1=→"Writing":i32)
              n1380 = call "IMAQ AVI Read Frame"("error in (no error)"=w316, "Frame Number"=w317, "Image"=w311, "Avi Refnum"=w310) -> ("error out"=w318:errorcluster, "Image Out"=w315:T2)  [unwired: 4 in, 2 out]
              n1381 = call "IMAQ AVI Write Frame"("error in (no error)"=w318, "Image"=w315, "Avi Refnum"=w312) -> ("error out"=w313:errorcluster, "Avi Refnum (duplicate)"=w314:T6)  [unwired: 7 in]
            }
            n1382 = call "IMAQ AVI Close"("error in (no error)"=w265, "Avi Refnum"=w266) -> ("error out"=w262:errorcluster)  [unwired: 9 in]
            n1383 = call "IMAQ Dispose"("Image"=w261, "error in (no error)"=w262) -> ("error out"=w249:errorcluster)  [unwired: 4 in]
            n1384 = case shown="False" w252 {
              tunnel: [string[] [] ("Video files to write") w290] -> w254
              tunnel: [i64[][] [] ("to write") w289] -> w253
              tunnel: ["Writing Complete" ("message") "Writing aborted" ("message")] -> w251
              tunnel: w250 -> [_ w287]
              tunnel: w249 -> [_ w286]
              frame False {
              }
              frame True {
                n1385 = local read "Video files to write"() -> (w290:string[])
                n1386 = Delete(path (use dialog)=w287, error in=w286) -> ()  [unwired: 3 in, 3 out]
                n1387 = local read "frames to write"() -> (w289:i64[][])
                n1388 = local write "Abort"(FALSE ("Abort")) -> ()
              }
            }
          }
          n1389 = One Button Dialog(message=w236) -> ()  [unwired: 1 in, 1 out]
          n1390 = local write "Video files to write"(w238) -> ()
          n1391 = local write "frames to write"(w237) -> ()
          n1392 = property on="Add to lib" class="Bool (strict)"("DisabledEnum"=w235) -> ()  [unwired: 2 in, 2 out]
          n1393 = property on="File name" class="Str"("DisabledEnum"=w235) -> ()  [unwired: 2 in, 2 out]
          n1394 = property on="Video to write" class="Path"("DisabledEnum"=w235) -> ()  [unwired: 2 in, 2 out]
          n1395 = property on="START" class="Bool (strict)"("DisabledEnum"=w235) -> ()  [unwired: 2 in, 2 out]
        }
      }
      n1396 = local read "START"() -> (w218:bool)
      n1397 = local write "Write file"(w225) -> ()
      n1398 = local write "Writing"(w219) -> ()
      n1399 = Wait (ms)(milliseconds to wait=u32 200) -> ()  [unwired: 1 out]
    }
    n1400 = while {
      tunnel: [w184] -> w6
      tunnel: w1 -> [_]
      stop <- w184 continue-if-true
      n1401 = case shown="True" "REPORT" {
        frame False {
        }
        frame True {
          w208 = TRUE ("open new instance (false)")
          n1402 = local read "Data file"() -> (w194:path)
          n1403 = local read "Video file"() -> (w193:path)
          n1404 = local write "REPORT"(FALSE ("REPORT")) -> ()
          n1405 = Strip Path(path=w194) -> (stripped path=w192:path)  [unwired: 1 out]
          n1406 = call <vilib>:"Get File Extension.vi"("file"=w193) -> ("filename without extension"=w189:string)  [unwired: 7 in, 3 out]
          n1407 = Path To String(path=w192) -> (string=w191:string)
          n1408 = Concatenate Strings(w191, "\\" ("string"), w189, " (BStAT Report).doc" ("string")) -> (w195:string)
          n1409 = String To Path(string=w195) -> (path=w197:path)
          n1410 = call <vilib>:"Check if File or Folder Exists.vi"("path"=w197) -> ("file or folder exists?"=w196:bool)  [unwired: 8 in, 2 out]
          n1411 = Automation Open(Automation Refnum=refnum<k7> refnum ("Word._Application"), 9:w208) -> (Automation Refnum=w201:refnum<k7>, error out=w202:errorcluster)  [unwired: 2 in]
          n1412 = property class="_Application"(reference=w201, error in=w202, "Visible"=w208) -> (reference out=w203:refnum<k7>, error out=w204:errorcluster)
          n1413 = case shown="True" w196 {
            tunnel: w197 -> [w211 w217]
            tunnel: [w210 w217] -> w187
            frame False {
              n1414 = Current VI's Path() -> (path=w214:path)
              n1415 = Strip Path(path=w214) -> (stripped path=w213:path)  [unwired: 1 out]
              n1416 = Build Path(base path=w213, name or relative path="BStAT report.doc") -> (appended path=w212:path)
              n1417 = One Button Dialog(message="***New report generated***\n\nRight-click on the white strip on the LEFT of the data area to copy the data ") -> ()  [unwired: 1 in, 1 out]
              n1418 = Copy(10:w211, 11:w212) -> (3:w210:path)  [unwired: 3 in, 2 out]
            }
            frame True {
              n1419 = One Button Dialog(message="***Report found***\n\nRight-click on the white strip on the LEFT of the data area to copy the data ") -> ()  [unwired: 1 in, 1 out]
            }
          }
          n1420 = property class="_Application"(reference=w203, error in=w204) -> (error out=w206:errorcluster, "Documents"=w205:refnum<k7>)  [unwired: 1 out]
          n1421 = invoke class="Documents" method="Open"(reference=w205, error in=w206, "FileName"=w187, "ReadOnly"=TRUE, "Visible"=TRUE) -> ()  [unwired: 14 in, 19 out]
        }
      }
      n1422 = local read "START"() -> (w184:bool)
      n1423 = Wait (ms)(milliseconds to wait=u32 200) -> ()  [unwired: 1 out]
    }
    n1424 = flat-sequence {
      tunnel: w7 -> [w33]
      tunnel: w6 -> [_]
      tunnel: w5 -> [_]
      tunnel: w4 -> [w34]
      frame #0 {
        w28 = T5 4 items=["Grayscale (U8)", "Grayscale (I16)", "Grayscale (SGL)", "Complex (CSG)", "RGB (U32)", "HSL (U32)", "RGB (U64)"] ("Image Type")
        w29 = T5 4 items=["Grayscale (U8)", "Grayscale (I16)", "Grayscale (SGL)", "Complex (CSG)", "RGB (U32)", "HSL (U32)", "RGB (U64)"] ("Image Type")
        w31 = T5 4 items=["Grayscale (U8)", "Grayscale (I16)", "Grayscale (SGL)", "Complex (CSG)", "RGB (U32)", "HSL (U32)", "RGB (U64)"] ("Image Type")
        n1425 = call "IMAQ AVI Close"("Avi Refnum"=w34) -> ("error out"=w32:errorcluster)  [unwired: 10 in]
        n1426 = Close File(refnum=w33, error in=w32) -> (error out=w26:errorcluster)  [unwired: 1 out]
        n1427 = call "IMAQ Create"("Image Name"="Video", "Image Type"=w28, "error in (no error)"=w26) -> ("New Image"=w22:T2, "error out"=w25:errorcluster)  [unwired: 2 in]
        n1428 = call "IMAQ Create"("Image Name"="pauselag", "Image Type"=w31, "error in (no error)"=w25) -> ("New Image"=w21:T2, "error out"=w23:errorcluster)  [unwired: 2 in]
        n1429 = call "IMAQ Create"("Image Name"="write", "Image Type"=w29, "error in (no error)"=w23) -> ("New Image"=w20:T2, "error out"=w19:errorcluster)  [unwired: 2 in]
        n1430 = call "IMAQ Dispose"("Image"=w22, "error in (no error)"=w19) -> ("error out"=w18:errorcluster)  [unwired: 4 in]
        n1431 = call "IMAQ Dispose"("Image"=w21, "error in (no error)"=w18) -> ("error out"=w17:errorcluster)  [unwired: 4 in]
        n1432 = call "IMAQ Dispose"("Image"=w20, "error in (no error)"=w17) -> ()  [unwired: 4 in, 1 out]
      }
    }
    n1433 = Wait (ms)(milliseconds to wait=u32 100) -> ()  [unwired: 1 out]
  }
